vi "Main2000.vi"() -> ()   [LabVIEW 2016]
doc: "Use this template to create an application that executes until you click the Stop button. Unlike the Single Loop Application VI that uses polling, this VI uses the Event Structure."
uses:
  <vilib>/vision/driver/NI_Vision_Acquisition_Software.lvlib
  <vilib>/vision/NI_Vision_Development_Module.lvlib
  Granule-2000AT/PC/llb/Library.lvlib
  <vilib>/Utility/file.llb/Write To Spreadsheet File (string).vi
  <vilib>/Utility/file.llb/Read From Spreadsheet File (string).vi
  <vilib>/userdefined/High Color/IMAQdx.ctl
panel:
  in  "Arhive":bool
  in  "M_PLasmatron":dbl
  out "V барабаны 2":dbl
  in  "Tab Control 2":enum32{"X1", "X2", "Y"}(tab)
  out "X240":bool[](array[boolean])
  out "ОП1 Х1 5":string[](array[string])
  out "X200":bool[](array[boolean])
  out "ОП1 Х1 4":string[](array[string])
  out "X140":bool[](array[boolean])
  out "ОП1 Х1 3":string[](array[string])
  out "X100":bool[](array[boolean])
  out "ОП1 Х1 2":string[](array[string])
  out "X400":bool[](array[boolean])
  out "ОП1 Х1 8":string[](array[string])
  out "X340":bool[](array[boolean])
  out "ОП1 Х1 7":string[](array[string])
  out "X300":bool[](array[boolean])
  out "ОП1 Х1 6":string[](array[string])
  out "Y120":bool[](array[boolean])
  out "ОП1 Х1 10":string[](array[string])
  out "Y60":bool[](array[boolean])
  out "ОП1 Х1 9":string[](array[string])
  out "Air 4":bool
  in  "PT3 2":dbl
  in  "Запись отчета":bool
  out "V вращ. бараб 2":string caption="V заготовки"
  out "LONGITUDINAL SPEED":string
  out "PLASMATRON SPEED":string
  in  "mac3":bool
  in  "Ошибка 2":i16 format="%x"
  in  "Скорость пп 2":i16
  out "Полож заг сер":bool
  out "Полож заг нач":bool caption="НАЧАЛО"
  out "Полож заг кон":bool
  out "Полож плазм кон":bool caption="Конец"
  out "Полож плазм сер":bool caption="Пром."
  out "Полож плазм  нач":bool caption="Начало"
  in  "МАКСИМАЛЬНАЯ СКОРОСТЬ ПП К":bool
  in  "v4066_cкорость подачи плазматрона":dbl
  in  "v4065_cкорость подачи":dbl
  in  "V7045_I_ist":dbl
  in  "V7045_U_ist":dbl
  in  "Действующий ток на плазматроне":string caption="Ток А"
  out "V заготовки":string
  in  "D, заготовки":i16
  in  "Закончить автораспыление":bool
  in  "Автораспыление доплавить":bool
  in  "Автораспыление начать":bool
  in  "задание тока А":string caption="Задание, А"
  in  "ПОДАЧА ЗАГОТОВКИ":bool
  in  "stop 3":bool
  in  "stop 2":bool
  in  "SP_зазор":dbl
  in  "PV_зазор":dbl
  in  "max out":dbl
  in  "out":dbl
  out "Distance зазор":sgl format="%.2f"
  out "x/y":dbl
  out "x*y":dbl
  out "16bit integer":i16
  in  "Numeric":i16
  in  "Т6":dbl
  in  "Улавливатель закрыть":bool
  in  "Улавливатель открыть":bool
  in  "Ролик прижать":bool
  in  "Ролик отжать":bool
  in  "PE3":dbl
  in  "PE2":dbl
  in  "PE1":dbl
  in  "ЗАДАНИЕ ТОКА":i16
  in  "ГС - Закрыть":bool
  in  "ГС -Открыть":bool
  out "ГС - Плазматрон":string caption="Плазматрон"
  out "ГС - Камера":string caption="Камера"
  in  "Скорость пп":i16
  in  "V барабаны задание":dbl
  in  "Выход":bool
  in  "ГС ПТ":i16
  in  "ГС камера":i16
  in  "V барабаны":dbl
  in  "Т5":dbl
  in  "Т4":dbl
  in  "Т3":dbl
  in  "Т2":dbl
  in  "Т1":dbl
  in  "Ошибка":i16
  in  "PT3":dbl
  in  "PT2":dbl
  in  "PT1":dbl
  in  "y120":i32
  in  "y60":i32
  in  "x400":i32
  in  "x340":i32
  in  "x300":i32
  in  "x240":i32
  in  "x200":i32
  in  "x140":i32
  in  "x100":i32
  in  "Tab Control":enum32{"VACUUM", "WORK", "INPUTS"}(tab)
  in  "forvacuum":bool
  in  "forvakuum led":bool
  in  "Slide":dbl(slide) scale=0.0..99.0
  out "PD2":u16(ring)
  out "NL 2":u16(ring)
  out "VP6":u16(ring)
  in  "ND HEAT BUT":bool
  in  "ND HEAT LED":bool
  in  "откачка стоп 2":bool
  in  "откачка стоп индик 2":bool
  out "Water-2":bool
  out "Water-1":bool
  out "Air":bool
  out "PT 4":string caption="Вакуум в камере\nPT2 (torr)"
  in  "откачка стоп":bool
  in  "откачка стоп индик":bool
  out "EV1":u16(ring)
  out "EV2":u16(ring)
  out "EV3.3":u16(ring)
  out "EV3.2":u16(ring)
  out "PE2":u16(ring)
  out "PE2":string caption="Вакуум в камере\nPT2 (torr)"
  out "CO1":u16(ring)
  out "CO2":u16(ring)
  out "EV3.1":u16(ring)
  out "CO3":u16(ring)
  out "P1":u16(ring)
  out "PE1":u16(ring)
  out "PE1":string caption="Вакуум в камере\nPT2 (torr)"
  out "PE3":u16(ring)
  out "PE3":string caption="Вакуум в камере\nPT2 (torr)"
  out "VP1":u16(ring)
  out "VP2":u16(ring)
  out "PT3":u16(ring)
  out "PT2":u16(ring)
  out "PT 2":string caption="Вакуум в камере\nPT2 (torr)"
  out "VP3":u16(ring)
  out "VP5":u16(ring)
  out "PD1":u16(ring)
  out "PT1":u16(ring)
  out "PT 1":string caption="Вакуум в камере\nPT2 (torr)"
  out "NZ":u16(ring)
  out "NB":u16(ring)
  out "NL":u16(ring)
  out "VP4":u16(ring)
  in  "mac 4":bool
  in  "напустить аргон":bool
  in  "откачать рабочий вакуум":bool
  in  "mac 2":bool
  out "PT 3":string caption="Вакуум в камере\nPT2 (torr)"
  out "УГ_закрыт":bool caption="Close"
  out "УГ_открыт":bool caption="Open"
  out "ролик_отжат":bool caption="Up"
  out "ролик_прижат":bool caption="Down"
  out "max Speed":string caption="Max speed (r/min)"
  out "ТЕМП КАМЕРА":string caption="T gas (C°)"
  in  "Скорость ПП 2":string caption="Plasmatron speed (mm/min)"
  in  "Скорость ПП":string caption="Longitudial speed (mm/min)"
  out "ТЕМП РОЛИК":string caption="T roller (C°)"
  out "ПОДШ. 2.2":string caption="T4 (C°)"
  out "ПОДШ. 2.1":string caption="T3 (C°)"
  out "ПОДШ. 1.2":string caption="T2 (C°)"
  out "ПОДШ. 1.1":string caption="T1 (C°)"
  out "P plasmatron (bar)":string
  out "P camera (bar)":string
  out "I_ist":string caption="Current (A)"
  out "U_ist":string caption="Voltage (V)"
  in  "Tab Control 3":enum32{"PARAMETERS VIDEO", "RID"}(tab)
  in  "Media Stop Button":bool
  in  "Play Button":bool
  in  "CAM":T1
  in  "HOOK":T2 {"Rotation" format="%.2f"; "Left" scale=0.0..1024.0; "Right" scale=0.0..1280.0}
  in  "PARAMETERS VIDEO":T3={"Contrast"=40, "Filter width"=4, "Steepness"=2, "Subsampling Ratio"=5, "Show Search Area"=FALSE, "Show Search Lines"=FALSE, "Show Edges Found"=FALSE, "Show Result"=TRUE}
  in  "WORK COLOR":u32(colorbox)
  in  "CALIBRATION":u32(colorbox)
  in  "DELAY":u32
  in  "BINAR LEVEL":cluster{"DOWN LEVEL":sgl, "UP LEVEL":sgl}={"DOWN LEVEL"=128.0, "UP LEVEL"=255.0} {"UP LEVEL" format="%.2f"; "DOWN LEVEL" format="%.2f"}
  in  "SHEMA":i32(ring)=1 items=["Red", "Green", "Blue", "Hue", "Saturation", "Luminance", "Value", "Intensity"]
  out "Индикатор камеры":bool
  in  "Blank Button":bool
  out "Индикатор камеры 2":bool
  in  "Сохранить настройки":bool
  out "String":string
  out "Record":bool
  out "Максимальная подача (мм/мин)2":string caption="Max speed\n(mm/min)"
  out "Boolean":bool
  in  "Регулятор":bool caption="RID"
  out "Actual speed\n(mm/min)":string
  out "PV(mm)":string
  out "SP (mm)":string
  in  "взять зазор":bool caption="Регулятор"
  out "Марка сплава":string caption="Mark"
  out "Порядковый номер":string caption="Billet number (un)"
  in  "Position (mm)":dbl(slide) scale=0.0..820.0
  out "Диаметр заг.":string caption="Diameter (mm)"
  out "V задания":string caption="Rotation speed (r/min)"
  out "V вращ. бараб":string caption="Rotation frequency (r/min)"
  in  "ЗУ-вверх":bool
  out "ИНдикатор положения полки":string
  in  "Продол впер":bool
  in  "Продол назад":bool
  in  "ПЛАЗМАТРОН В ИСХОДНОЕ":bool
  out "индикация видео":T4(plugin-control)
  in  "ПЛАЗМАТРОН В ИСХОДНОЕ 2":bool
  out "PULLEYS":dbl(graph)
  out "PV":dbl(graph)
  out "LONGITUDINAL FEED":dbl(graph)
  out "CURRENT":dbl(graph)
  out "VOLTAGE":dbl(graph)
  out "voto plasmatron":string caption="MOTO\nPLASMATRON"
  out "текущее время":string
  # "Ролик"
  # "Улавливатель ОГ"
  # "Обработка"
  # "БАРАБАНЫ"
  # "РАСПЫЛЕНИЕ ЗАГОТОВКИ"
  # "Температура"
  # "3A3.1 X100-X137"
  # "3A3.2 X140-177"
  # "3A4 X200-X237"
  # "3A5.1 X240-X277"
  # "3A5.2 X300-X337"
  # "3A6 X340-X377"
  # "3A8 X400-X437"
  # "2A8 Y60-Y117"
  # "3A7 Y120-Y157"
  # "Положение толкателя"
  # "Положение плазматрона"
  # "Газовая система"
  # "VF1"
  # "Ar,He"
  # "PC1"
  # "PC2"
  # "SYSTEM"
  # "PLASMATRON"
  # "CATCHER CINDERS"
  # "PINCH ROLLER"
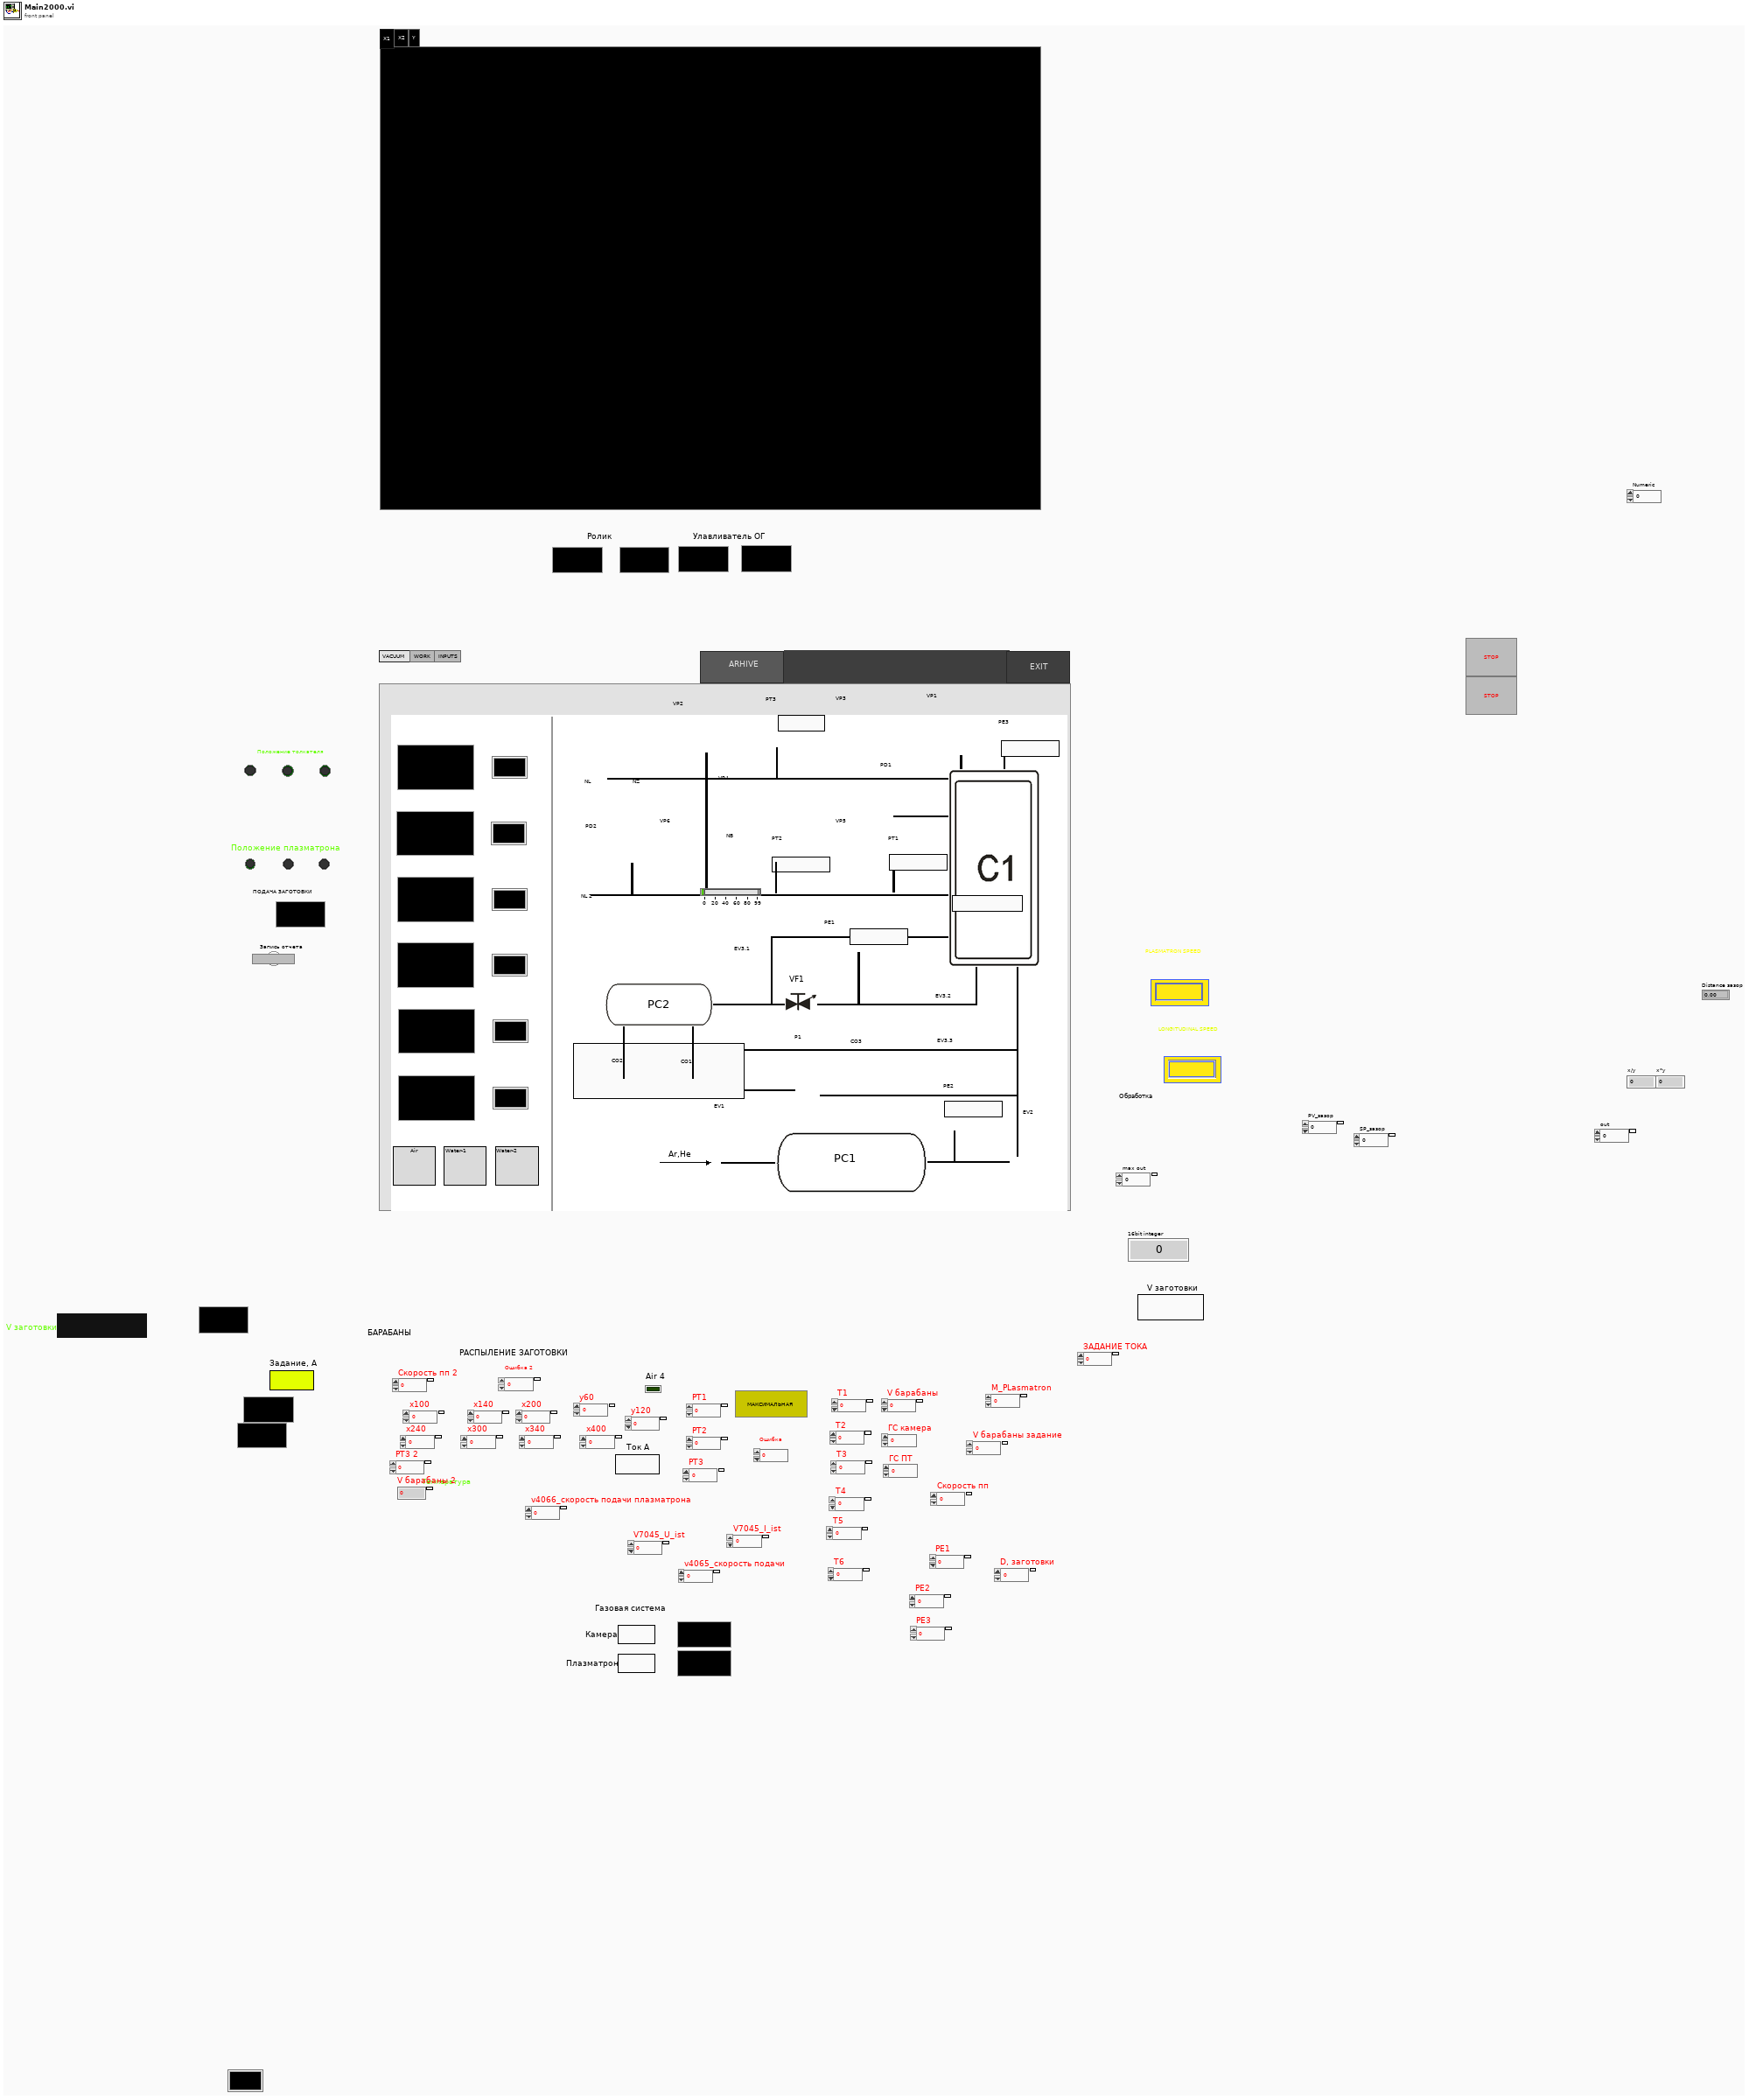
[diagram p1: front panel]
types:
  T1 = typedef "Library.lvlib/IMAQdx.ctl" = refnum<k21>
  T2 = typedef "IMAQ Rectangle" = cluster{"Left":i32, "Top":i32, "Right":i32, "Bottom":i32, "Rotation":dbl}
  T3 = cluster{"Contrast":i32, "Filter width":i32, "Steepness":i32, "Subsampling Ratio":u32, "Show Search Area":bool, "Show Search Lines":bool, "Show Edges Found":bool, "Show Result":bool}
  T4 = typedef "IMAQ Image.ctl" = refnum<image>
  T5 = enum16{"open", "replace", "create", "open or create", "replace or create", "replace or create with confirmation"}
  T6 = enum8{"Enabled", "Disabled", "Disabled and Grayed Out"}
  T7 = cluster{i32, i32, i32, u32, "Boolean":bool, "Boolean":bool, "Boolean":bool, "Boolean":bool}
  T8 = typedef "Image Type" = u32
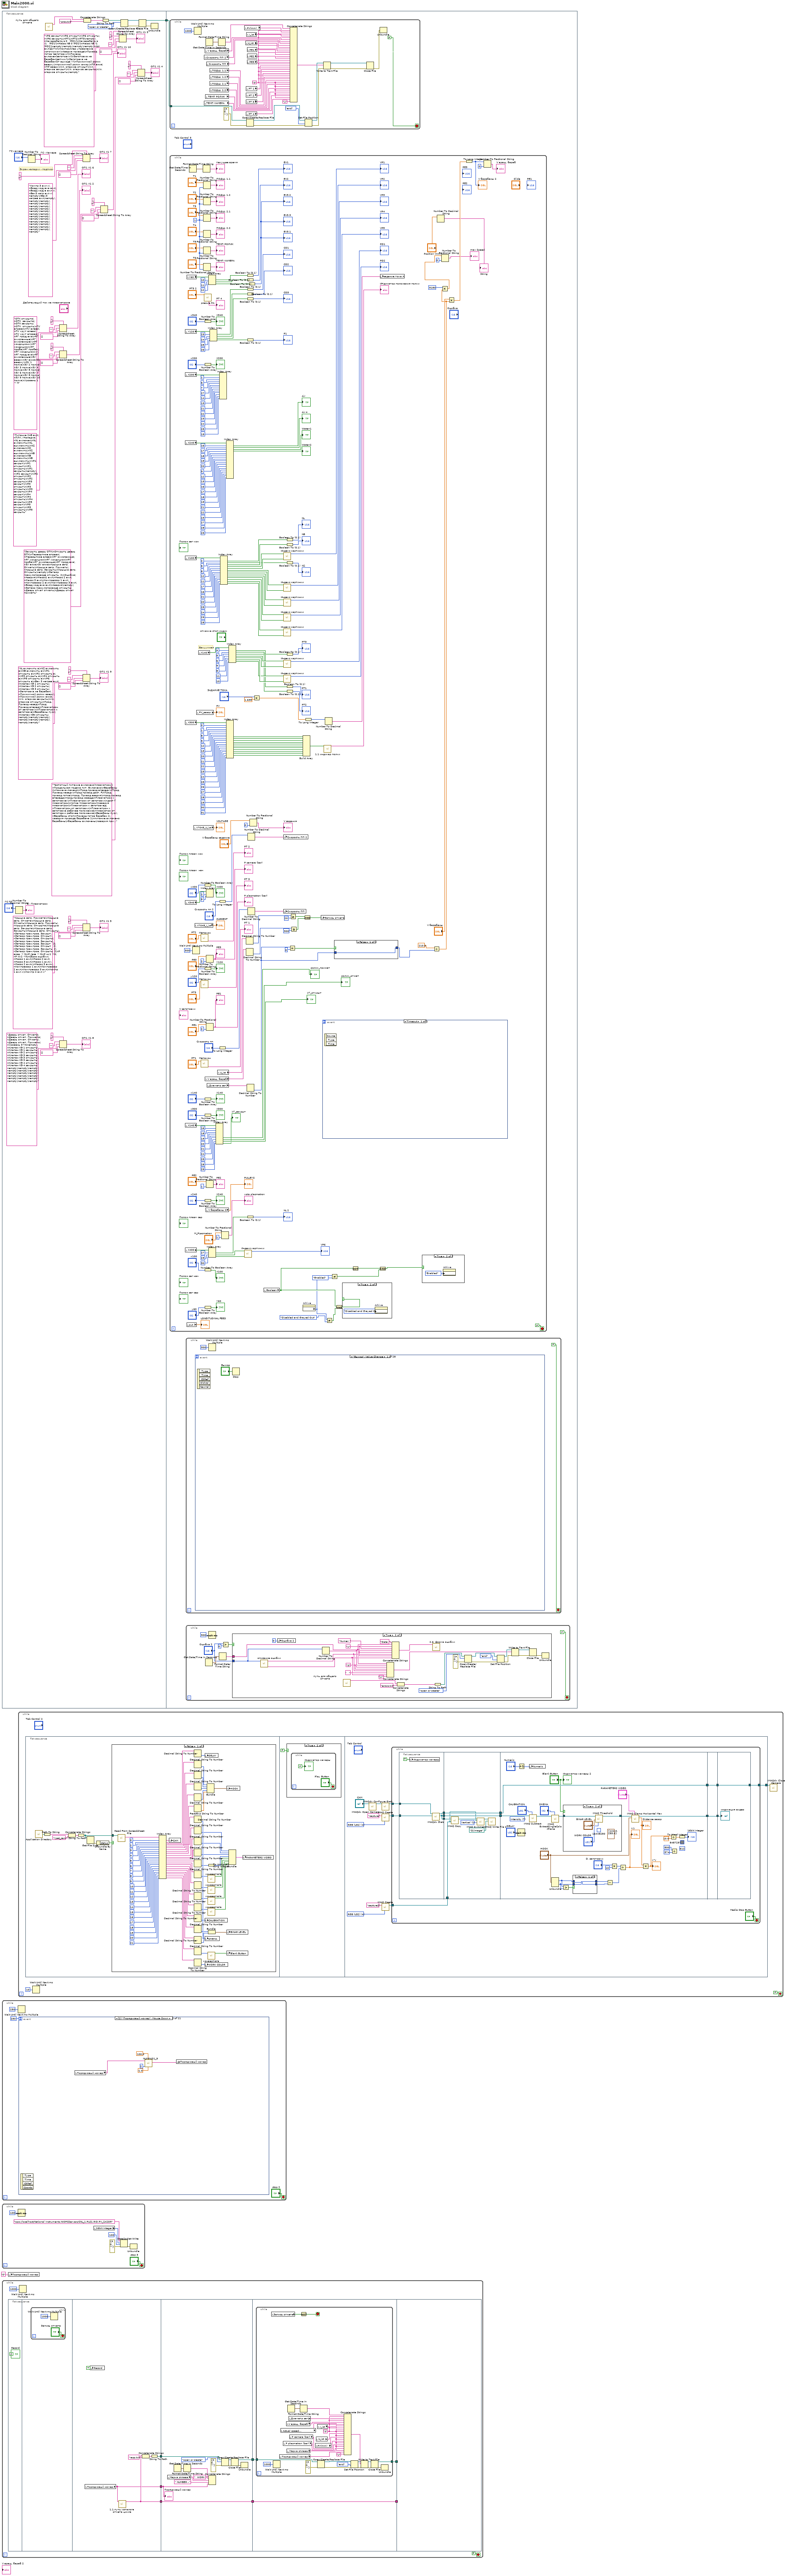
[diagram p0: block diagram]
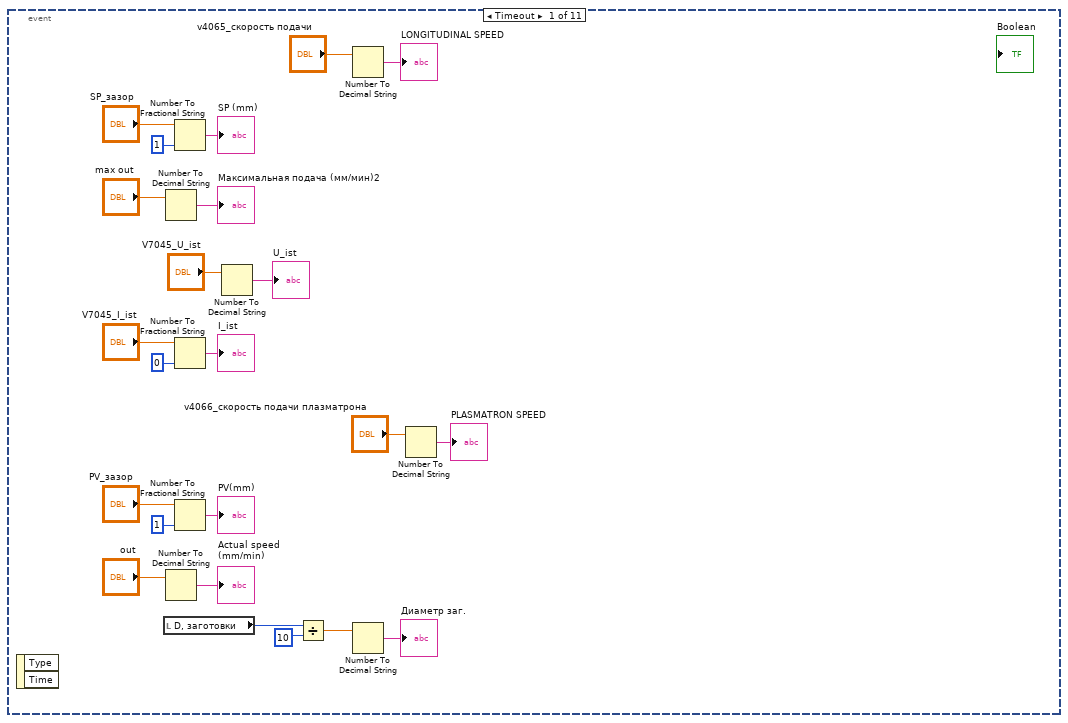
[diagram p6: hidden frame]
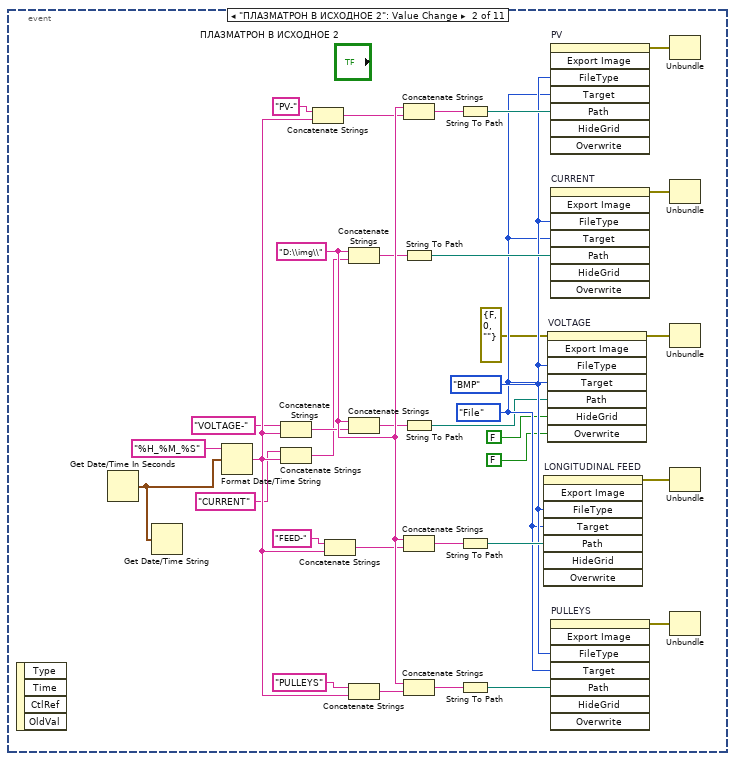
[diagram p7: hidden frame]
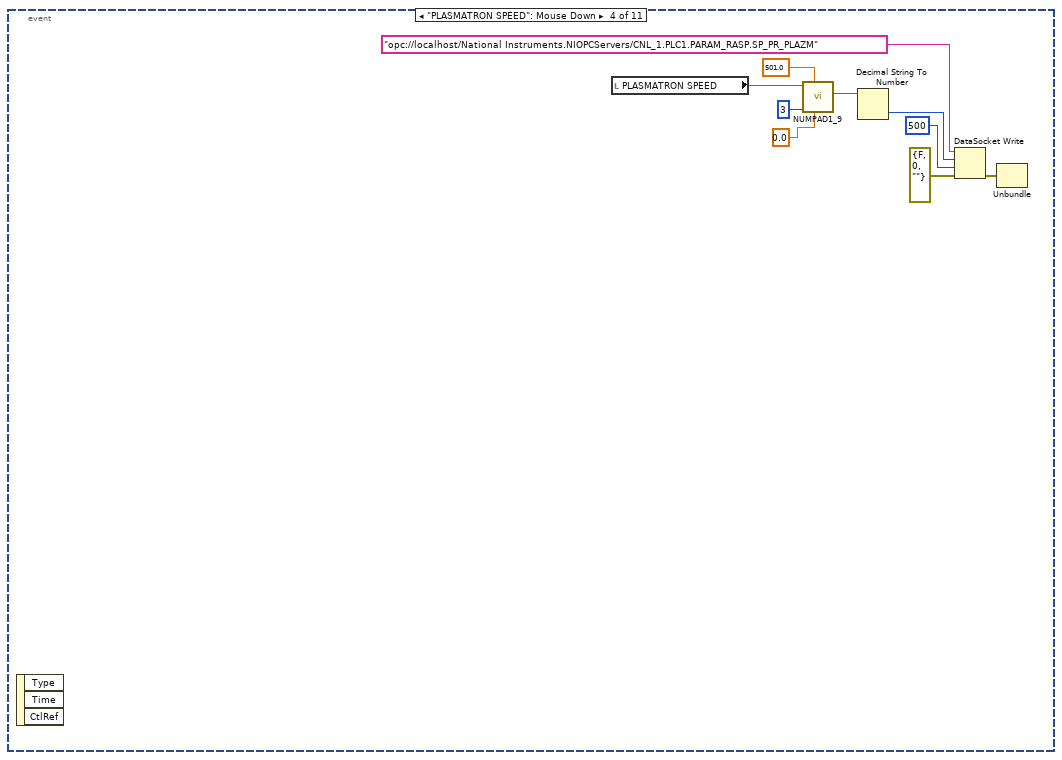
[diagram p8: hidden frame]
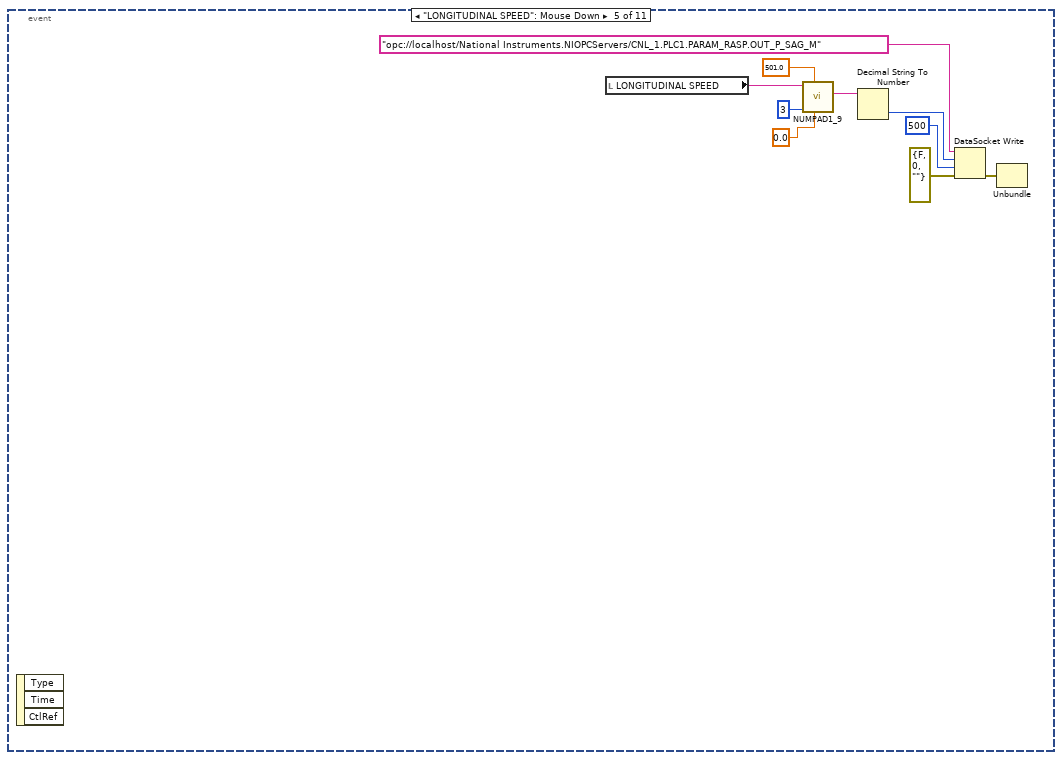
[diagram p9: hidden frame]
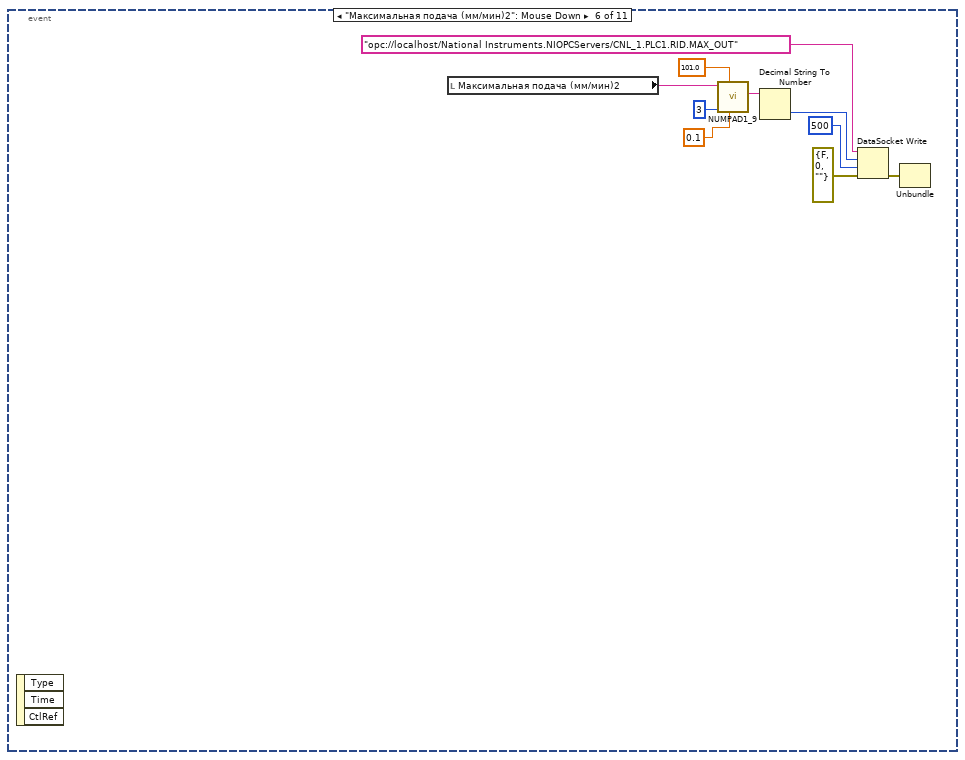
[diagram p10: hidden frame]
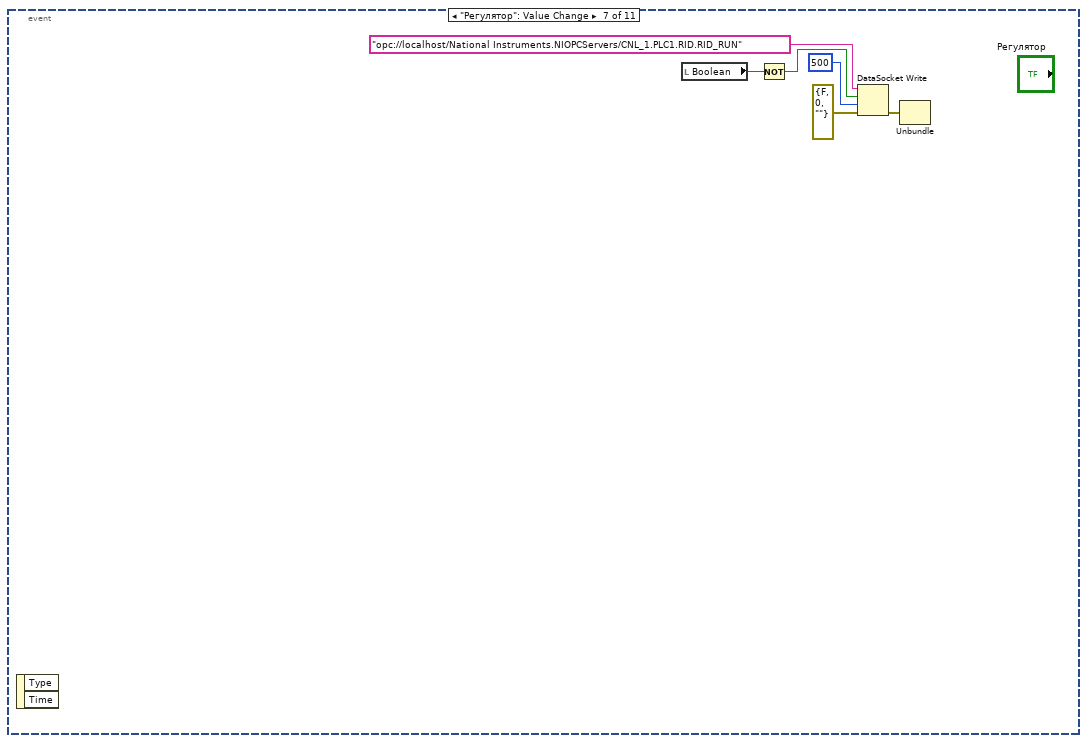
[diagram p11: hidden frame]
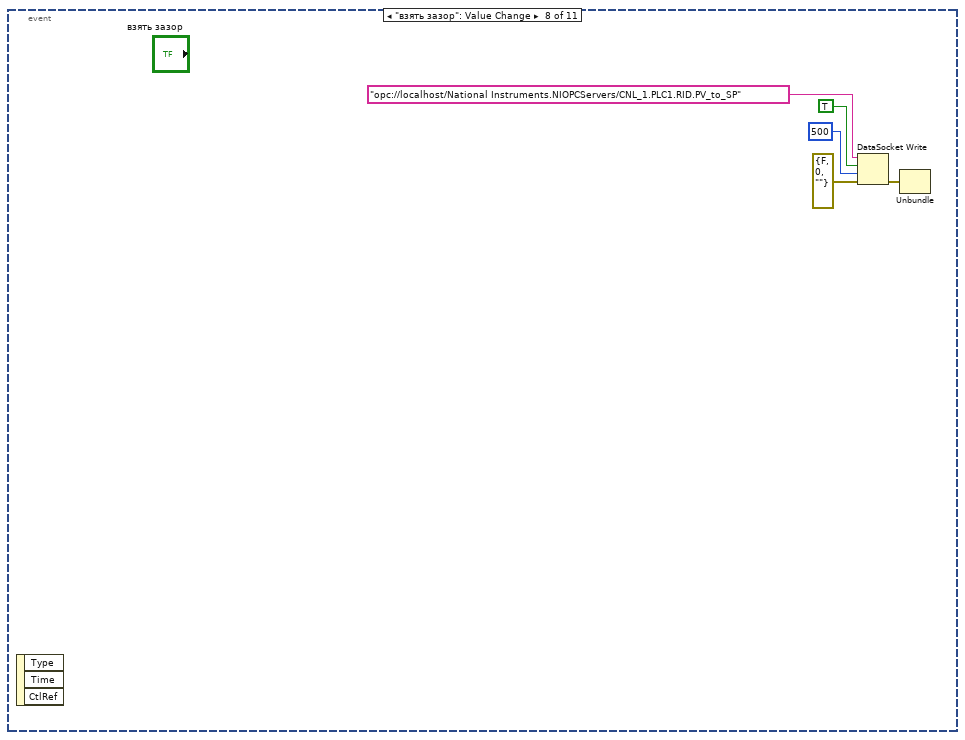
[diagram p12: hidden frame]
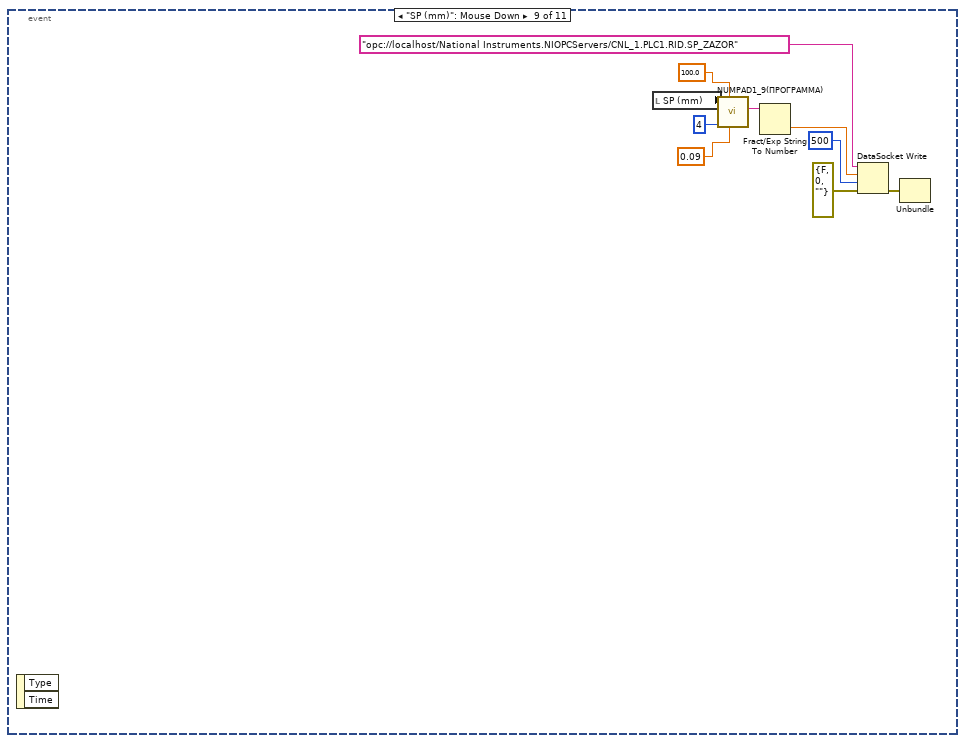
[diagram p13: hidden frame]
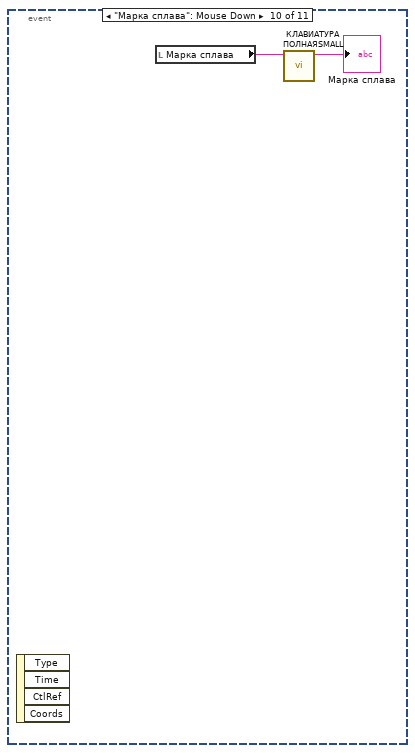
[diagram p14: hidden frame]
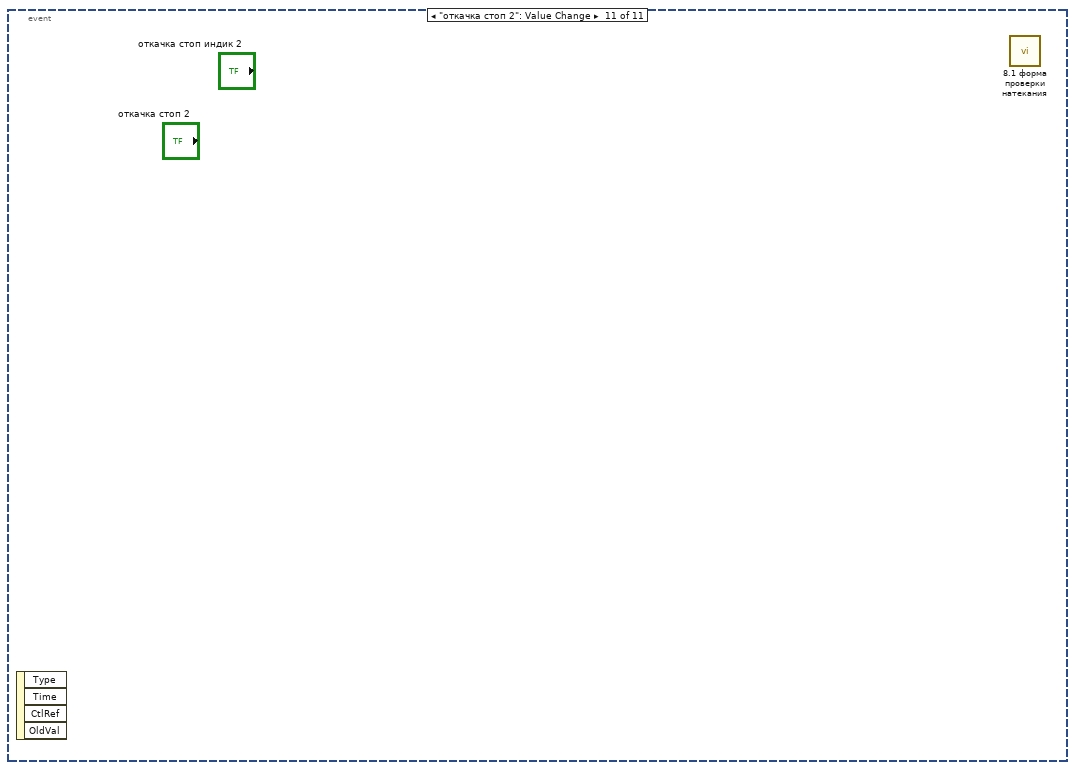
[diagram p15: hidden frame]
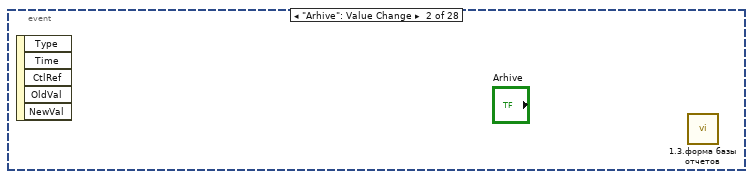
[diagram p17: hidden frame]
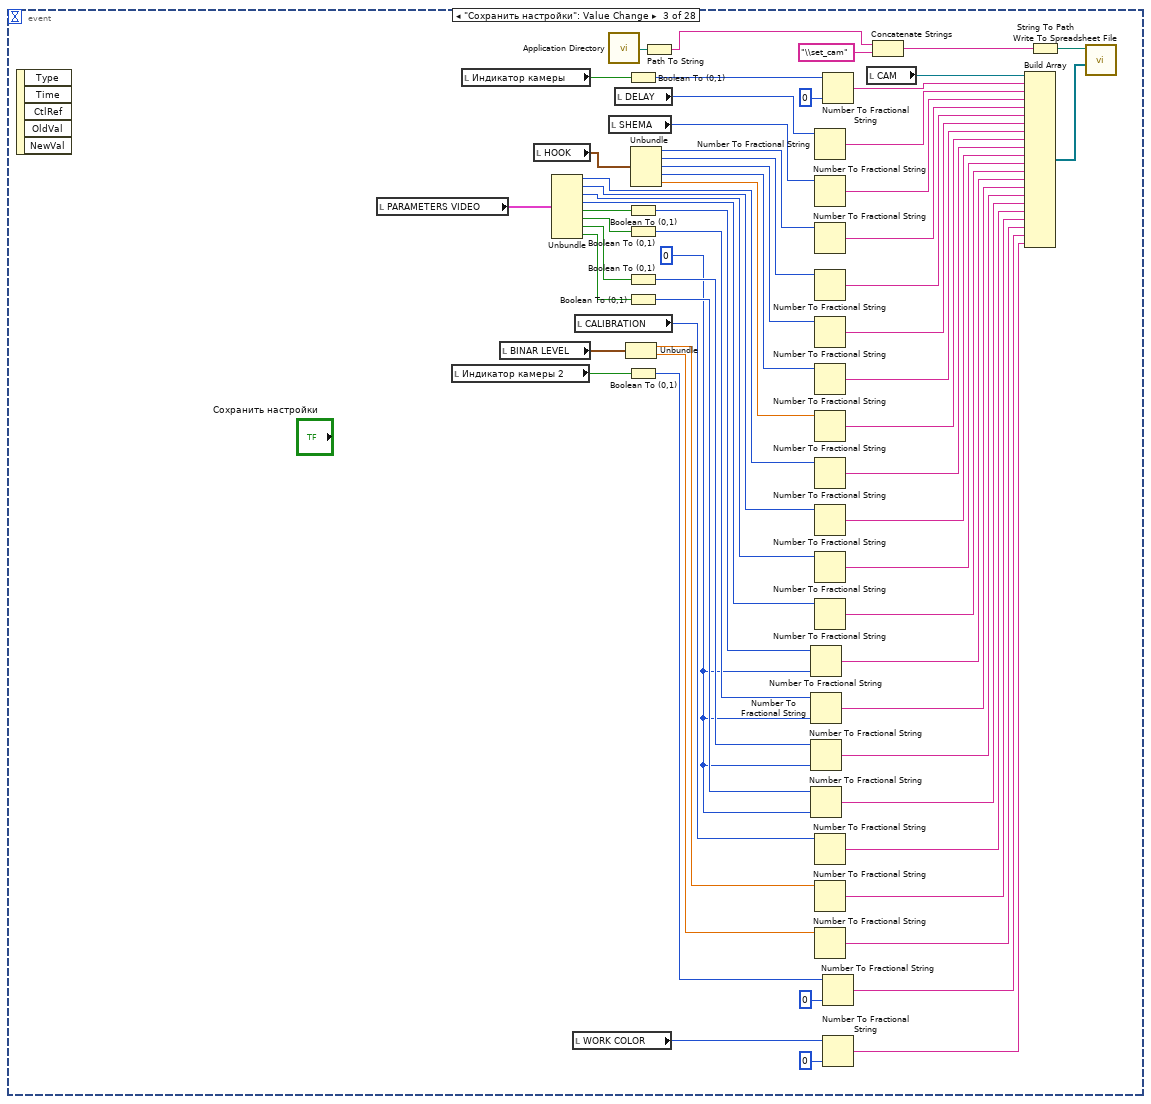
[diagram p18: hidden frame]
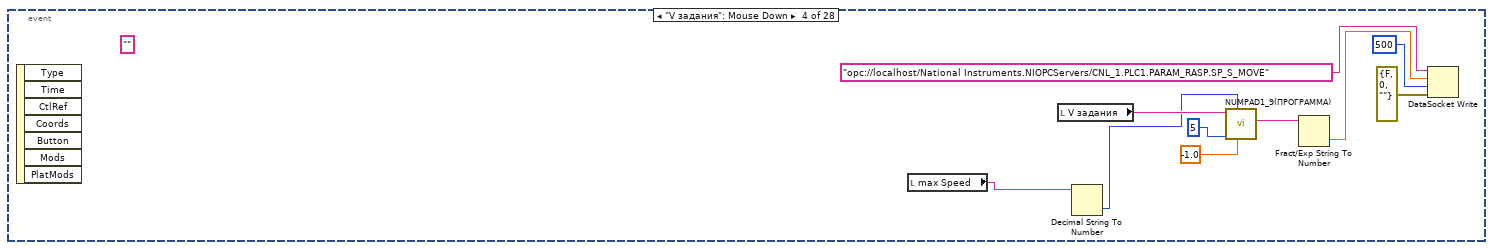
[diagram p19: hidden frame]
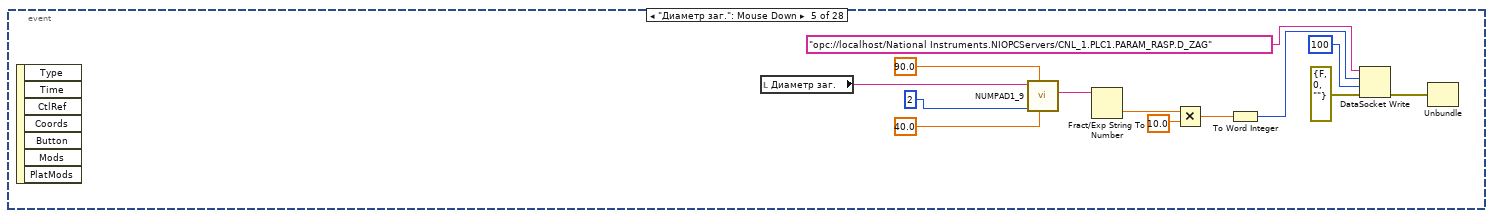
[diagram p20: hidden frame]
diagram:
  n1 = flat-sequence {
    tunnel: [w3] -> w1
    tunnel: w1 -> [w61]
    frame #0 {
      # "Экран наладки - подписи"
      n2 = Number To Decimal String(number="ГС ПТ") -> (decimal integer string=→"ГС - Плазматрон":string)  [unwired: 1 in]
      n3 = Number To Decimal String(number="ГС камера") -> (decimal integer string=→"ГС - Камера":string)  [unwired: 1 in]
      n4 = call "путь для общего отчета.vi"() -> ("path_out 2"=w9:string)  [unwired: 11 in]
      n5 = Spreadsheet String To Array(delimiter (Tab)="\n", format string="", spreadsheet string="ОТК открыта\nОТК  закрыта\nОТК закрыть\nОТК  открыть\nПУ вправо\nПУ влево\nПУ крут влево\nПУ крут вправо\nРГ продувка\nРГ окисленные\nРГ окисленныек\nРГ кондиционк\nРГ кондицион\nРГ проба\nРГ пробак\nРГ кондиционкк\nРГ продувка\nРГ окисленные\nЗУ вверх\nЗУ вниз\nЗУ вверху\nЗУ 1 полка\nЗУ 2 полка\nЗУ 3 полка\nЗУ 4 полка\nЗУ 5 полка\nЗУ 6 полка\nЗУ 7 полка\nЗУ 8 полка\nЗУ 9 полка\nЗУ 10 полка\nУровень 1 < N", array type (2D Dbl)=string[] [] ("ОП1 Х1")) -> (array=→"ОП1 Х1 6":string[])
      n6 = Spreadsheet String To Array(delimiter (Tab)="\n", format string="", spreadsheet string="Питание 24В вкл\nПЛК / Наладка\nNL включен\nNL включить\nNL выключить\nNZ включен\nNZ включить\nNZ выключить\nNB включен\nNB включить\nNB выключить\nVP1 закрыт\nVP1 открыт\nVP1 открыть\nVP1 закрыть\nempty\nVP2 закрыт\nVP2 открыт\nVP2 открыть\nVP2 закрыть\nVP3 закрыт\nVP3 открыт\nVP3 открыть\nVP3 закрыть\nVP4 закрыт\nVP4 открыт\nVP4 открыть\nVP4 закрыть\nVP5 закрыт\nVP5 открыт\nVP5 открыть\nVP5 закрыть", array type (2D Dbl)=string[] [] ("ОП1 Х1")) -> (array=→"ОП1 Х1 2":string[])
      n7 = Spreadsheet String To Array(delimiter (Tab)="\n", format string="", spreadsheet string="Дверь откат. Отжата\nДверь откат. Прижата\nДверь откат. Отжать\nДверь откат. Прижать\nУровень 3<N\nempty\nКлапан КЭ 1 открыть\nКлапан КЭ 1 закрыть\nКлапан КЭ 2 открыть\nКлапан КЭ 3 закрыть\nКлапан КЭ 3 открыть\nКлапан КЭ 3 закрыть\nКлапан КЭ 4 открыть\nКлапан КЭ 4 закрыть\nempty\nempty\nempty\nempty\nempty\nempty\nempty\nempty\nempty\nempty\nempty\nempty\nempty\nempty\nempty\nempty\nempty\nempty", array type (2D Dbl)=string[] [] ("ОП1 Х1")) -> (array=→"ОП1 Х1 8":string[])
      n8 = Spreadsheet String To Array(delimiter (Tab)="\n", format string="", spreadsheet string="Компр 3 вкл к\nВоздуходувка вкл\nВоздуходув вкл к\nБак3 нагр вкл к\nempty\nБак3 нагрев вкл\nempty\nempty\nempty\nempty\nempty\nempty\nempty\nempty\nempty\nempty\nempty\nempty\nempty\nempty\nempty\nempty\nempty\nempty\nempty\nempty\nempty\nempty\nempty\nempty\nempty\nempty", array type (2D Dbl)=string[] [] ("ОП1 Х1")) -> (array=→"ОП1 Х1 7":string[])
      n9 = Spreadsheet String To Array(delimiter (Tab)="\n", format string="", spreadsheet string="NL включить в\nNZ включить в\nNB включить в\nVP1 открыть в\nVP2 открыть в\nVP3 открыть в\nVP4 открыть в\nVP5 открыть в\nVP6 открыть в\nБак 3 нагрев вкл\nКлапан КЭ 1 открыть\nКлапан КЭ 2 открыть\nКлапан КЭ 3 открыть\nЗаготовка на барабан\nПрижимной ролик вверх\nПрижимной ролик вниз\nУл. огарков закрыть\nУл. огарков открыть\nПрод. Привод назад\nПрод. Привод вперед\nПлазматрон от заготовки\nПлазматрон к заготовке\nБарабаны пуск\nКлапан КЭ4 открыть\nempty\nempty\nempty\nempty\nempty\nempty\nempty\nempty", array type (2D Dbl)=string[] [] ("ОП1 Х1")) -> (array=→"ОП1 Х1 9":string[])
      n10 = Spreadsheet String To Array(delimiter (Tab)="\n", format string="", spreadsheet string="Крышка загр. Прижата\nКрышка загр. Отжата\nКрышка загр. Отжать\nКрышка загр. Прижать\nКрышка загр. Открыта\nКрышка загр. Закрыта\nКрышка загр. Закрыть\nКрышка загр. Открыть\nЗатвор гран.пров. Закрыт\nЗатвор гран.пров. Открыт\nЗатвор гран.пров. Открыть\nЗатвор гран.пров. Закрыть\nЗатвор гран.пров. Закрыт   2\nЗатвор гран.пров. Открыт   2\nЗатвор гран.пров. Закрыть  2\nЗатвор гран.пров. Открыть  2\nP возд. < N\nP газа < N\nP нк1 <N\nP нк2 <N\nСброс ошибки\nНасос 1 вкл\nНасос 2 вкл\nНасос 3 вкл\nНасос 1 вклк\nНасос 2 вклк\nНасос 3 вклк\nКомпрессор 1 вкл\nКомпрессор 2 вкл\nКомпрессор 3 вкл\nКомпр 1 вкл к\nКомпр 2 вкл к", array type (2D Dbl)=string[] [] ("ОП1 Х1")) -> (array=→"ОП1 Х1 5":string[])
      n11 = Concatenate Strings(w9, "proc.txt") -> (w11:string)
      n12 = Spreadsheet String To Array(delimiter (Tab)="\n", format string="", spreadsheet string="Закрыть дверь ОТК\nОткрыть дверь ОТК\nПересыпное вправо\nПересыпное влево\nРГ окисленные\nРГ кондицион\nРГ кондицион\nРГ проба\nРГ окисленные\nРГ продувка\nЗУ вниз\nЗУ вниз\nКрышка загр. Отжать\nКрышка загр. Прижать\nКрышка загр. Закрыть\nКрышка загр. Открыть\nempty\nЗатвор гранулопровода открыть  2\nОшибка\nАвария\nНасос1 вкл\nНасос 2 вкл\nНасос 3 вкл\nКомпрессор 1 вкл\nКомпрессор 2 вкл\nКомпрессор 3 вкл\nВоздуходувка вкл\nАвария\nempty\nЗатвор гранулопровода открыть\nДверь откат отжать\nДверь откат прижать", array type (2D Dbl)=string[] [] ("ОП1 Х1")) -> (array=→"ОП1 Х1 10":string[])
      n13 = String To Path(string=w11) -> (path=w7:path)
      n14 = Spreadsheet String To Array(delimiter (Tab)="\n", format string="", spreadsheet string="VP6 закрыт\nVP6 открыт\nVP6 открыть\nVP6 закрыть\nPT1\nPT2\nPT3\nempty\nКамераЗагруз 0   (PD1)\nКамераЗагруз -1   (PD1)\nНасос NB 0 (PD2)\nНасос NB -1 (PD2)\nempty\nempty\nempty\nempty\nИст вкл(ДУГА)\nКонтроллер управление источником\nАвария привода\nПривод готов (заготовки)\nПривод включен(заготовки)\nЗаготовка на барабан(датчик)\nЗаготовка на барабан(от выхода Y)\nПрижимной ролик вверху\nприжимной ролик внизу\nПР вниз\nПР вверх\nУл. огарков открыт\nУл. огарков закрыт\nУл. огарков закрыть\nУл. огарков открыть\nempty", array type (2D Dbl)=string[] [] ("ОП1 Х1")) -> (array=→"ОП1 Х1 3":string[])
      n15 = Open/Create/Replace File(file path (use dialog)=w7, operation (0:open)=T5."open or create") -> (refnum out=w4:refnum<file>, error out=w5:errorcluster)  [unwired: 4 in, 1 out]
      n16 = Spreadsheet String To Array(delimiter (Tab)="\n", format string="", spreadsheet string="Частотный питание включено(плазматрон)\nПродольная подача пит. Включено\nБарабаны питание включено\nПрод.привод впередк\nПрод. Привод назадк\nПрод привод дост. F\nПрод.привод готов\nпрод. Привод авария\nпрод.привод впередд\nпрод.привод назадд\nПлазматрон к заготовкек\nПлазматрон от заготовки\nдост f   плазматрон\nготов (плазматрон)\nавария плазматрон\nПлазматрон к заготовкед\nПлазматрон от заготовки\nПлазматрон к заготовке рабочее положение\nплазматро от заготовки рабочее положение\nБарабаны пуск\nБарабаны стоп\nПривод готов барабан 1\nавария привода барабана 1\nпитание включено барабаны\nбарабаны включены\nавария привода барабана 2\nпривод готов барабан 2\nПеремещение плазматрона пит. Включено\nempty\nПрижимной ролик вверху\nПрижимной ролик внизу\nempty", array type (2D Dbl)=string[] [] ("ОП1 Х1")) -> (array=→"ОП1 Х1 4":string[])
      n17 = Close File(refnum=w4, error in=w5) -> (path=w3:path, error out=w8:errorcluster)
      n18 = Unbundle(w8) -> ()  [unwired: 3 out]
    }
    frame #1 {
      n19 = while {
        tunnel: w61 -> [w88]
        stop <- FALSE stop-if-true
        w64 = "\t"
        n20 = Wait Until Next ms Multiple(millisecond multiple=u32 1000 ("milliseconds to wait")) -> ()  [unwired: 1 out]
        n21 = local read "Скорость ПП 2"() -> (w82:string)
        n22 = local read "ТЕМП КАМЕРА"() -> (w65:string)
        n23 = local read "V вращ. бараб"() -> (w83:string)
        n24 = local read "ТЕМП РОЛИК"() -> (w71:string)
        n25 = Get Date/Time In Seconds() -> (seconds since 1Jan1904=w97:timestamp)
        n26 = local read "Скорость ПП"() -> (w81:string)
        n27 = local read "ПОДШ. 1.1"() -> (w69:string)
        n28 = local read "ПОДШ. 1.2"() -> (w74:string)
        n29 = local read "ПОДШ. 2.1"() -> (w73:string)
        n30 = local read "ПОДШ. 2.2"() -> (w72:string)
        n31 = Format Date/Time String(seconds (now)=w97) -> (date/time string=w66:string)  [unwired: 2 in]
        n32 = local read "PV(mm)"() -> (w67:string)
        n33 = local read "U_ist"() -> (w80:string)
        n34 = local read "PT 1"() -> (w76:string)
        n35 = local read "PT 2"() -> (w75:string)
        n36 = local read "PT 3"() -> (w70:string)
        n37 = local read "PT 4"() -> (w63:string)
        n38 = local read "I_ist"() -> (w68:string)
        n39 = Open/Create/Replace File(file path (use dialog)=w88, error in=errorcluster {"status"=FALSE, "code"=0, "source"=""}) -> (refnum out=w96:refnum<file>, error out=w94:errorcluster)  [unwired: 4 in, 1 out]
        n40 = local read "PE1"() -> (w79:string)
        n41 = local read "PE2"() -> (w78:string)
        n42 = local read "PE3"() -> (w77:string)
        n43 = Concatenate Strings(w66, w64, w67, w64, w68, w64, w83, w64, w82, w64, w81, w64, w80, w64, w79, w64, w78, w64, w77, w64, w76, w64, w75, w64, w70, w64, w69, w64, w74, w64, w73, w64, w72, w64, w71, w64, w65, w64, w63, "\r") -> (w86:string)
        n44 = Set File Position(refnum=w96, from (0:start)=enum16{"start", "end", "current"}."end", error in=w94) -> (refnum out=w93:refnum<file>, error out=w92:errorcluster)  [unwired: 1 in]
        n45 = Write to Text File(file (use dialog)=w93, text=w86, error in=w92) -> (refnum out=w91:refnum<file>, error out=w90:errorcluster)  [unwired: 1 in, 1 out]
        n46 = Close File(refnum=w91, error in=w90) -> (error out=w89:errorcluster)  [unwired: 1 out]
        n47 = Unbundle(w89) -> ()  [unwired: 3 out]
      }
      n48 = while {
        stop <- FALSE stop-if-true
        w394 = i16 1 ("precision (6)")
        # "Вакуумная"
        n49 = local read "Y120"() -> (w544:bool[])
        n50 = local read "X200"() -> (w606:bool[])
        n51 = local read "X240"() -> (w590:bool[])
        n52 = local read "X100"() -> (w410:bool[])
        n53 = local read "X300"() -> (w565:bool[])
        n54 = local read "X340"() -> (w551:bool[])
        n55 = local read "X140"() -> (w625:bool[])
        n56 = local read "X400"() -> (w473:bool[])
        n57 = local read "Y60"() -> (w545:bool[])
        n58 = local read "out"() -> (→"LONGITUDINAL FEED":dbl)
        n59 = Get Date/Time In Seconds() -> (seconds since 1Jan1904=w483:timestamp)
        n60 = Wait Until Next ms Multiple(millisecond multiple=u32 500) -> ()  [unwired: 1 out]
        n61 = local read "V7045_U_ist"() -> (→"VOLTAGE":dbl)
        n62 = local read "V7045_I_ist"() -> (→"CURRENT":dbl)
        n63 = local read "PV_зазор"() -> (→"PV":dbl)
        n64 = local read "X140"() -> (w445:bool[])
        n65 = call "Метакон.vi"("Vak_in"="PT2") -> ("Vak_out_txt"=→"PT 2":string)  [unwired: 9 in, 1 out]
        n66 = call "Метакон.vi"("Vak_in"="PT3") -> ("Vak_out_txt"=→"PT 3":string)  [unwired: 9 in, 1 out]
        n67 = call "Метакон.vi"("Vak_in"="PT1") -> ("Vak_out_txt"=→"PT 1":string)  [unwired: 9 in, 1 out]
        n68 = Format Date/Time String(seconds (now)=w483) -> (date/time string=→"текущее время":string)  [unwired: 2 in]
        n69 = Number To Fractional String(number="Т1", precision (6)=w394) -> (F-format string=→"ПОДШ. 1.1":string)  [unwired: 2 in]
        n70 = Number To Fractional String(number="Т2", precision (6)=w394) -> (F-format string=→"ПОДШ. 1.2":string)  [unwired: 2 in]
        n71 = Number To Fractional String(number="Т3", precision (6)=w394) -> (F-format string=→"ПОДШ. 2.1":string)  [unwired: 2 in]
        n72 = Number To Fractional String(number="Т4", precision (6)=w394) -> (F-format string=→"ПОДШ. 2.2":string)  [unwired: 2 in]
        n73 = Number To Fractional String(number="Т5", precision (6)=w394) -> (F-format string=→"ТЕМП РОЛИК":string)  [unwired: 2 in]
        n74 = Number To Fractional String(number="Т6", precision (6)=w394) -> (F-format string=→"ТЕМП КАМЕРА":string)  [unwired: 2 in]
        n75 = call "presure PA.vi"("Volte"="PT3 2") -> ("presure String 2"=→"PT 4":string)  [unwired: 7 in, 3 out]
        n76 = Number To Boolean Array(number="x340") -> (Boolean array=→"X340":bool[])
        n77 = Number To Boolean Array(number="x200") -> (Boolean array=→"X200":bool[])
        n78 = Number To Boolean Array(number="x400") -> (Boolean array=→"X400":bool[])
        n79 = Number To Boolean Array(number="y120") -> (Boolean array=→"Y120":bool[])
        n80 = Number To Boolean Array(number="x140") -> (Boolean array=→"X140":bool[])
        n81 = Number To Boolean Array(number="x300") -> (Boolean array=→"X300":bool[])
        n82 = Number To Boolean Array(number="x240") -> (Boolean array=→"X240":bool[])
        n83 = Number To Boolean Array(number="x100") -> (Boolean array=→"X100":bool[])
        n84 = Number To Boolean Array(number="y60") -> (Boolean array=→"Y60":bool[])
        n85 = local read "V вращ. бараб"() -> (w510:string)
        n86 = local read "V барабаны 2"() -> (→"PULLEYS":dbl)
        n87 = Index Array(array=w551, index #1=2, index #2=5) -> ()  [unwired: 2 out]
        n88 = Number To Fractional String(number="PE3", precision (6)=i16 2) -> (F-format string=→"PE3" →"P camera (bar)":string)  [unwired: 2 in]
        n89 = Number To Fractional String(number="PE1", precision (6)=i16 2) -> (F-format string=→"PE1" →"P plasmatron (bar)":string)  [unwired: 2 in]
        n90 = Number To Fractional String(number="PE2", precision (6)=i16 1) -> (F-format string=→"PE2":string)  [unwired: 2 in]
        n91 = local read "Диаметр заг."() -> (w402:string)
        n92 = Index Array(array=w545, index #1=10, index #2=11, index #3=12) -> (element #1=w539:bool, element #2=w538:bool, element #3=w537:bool)
        n93 = Index Array(array=w473, index #1=27, index #2=29, index #3=30) -> (element #1=w477:bool, element #2=w480:bool, element #3=w481:bool)
        n94 = Index Array(array=w544, index #1=23, index #2=24, index #3=25, index #4=26) -> (element #1=w533:bool, element #2=w532:bool, element #3=w531:bool, element #4=w530:bool)
        n95 = Index Array(array=w625, index #1=16, index #2=18, index #3=19, index #4=20, index #5=21, index #6=24, index #7=25, index #8=28, index #9=29) -> (element #6=→"ролик_прижат":bool, element #7=→"ролик_отжат":bool, element #8=→"УГ_открыт":bool, element #9=→"УГ_закрыт":bool)  [unwired: 5 out]
        n96 = local read "U_ist"() -> (w505:string)
        n97 = To Long Integer(number="Скорость пп 2") -> (32bit integer=w399:i32)
        n98 = To Long Integer(number="Скорость пп") -> (32bit integer=w375:i32)
        n99 = Index Array(array=w606, index #1=1, index #2=6, index #3=7, index #4=27, index #5=14, index #6=13, index #7=21, index #8=22, index #9=23, index #10=24, index #11=25, index #12=19) -> ()  [unwired: 12 out]
        n100 = Index Array(array=w410, index #1=2, index #2=5, index #3=8, index #4=12, index #5=11, index #6=17, index #7=16, index #8=21, index #9=20, index #10=25, index #11=24, index #12=29, index #13=28) -> (element #1=w412:bool, element #2=w416:bool, element #3=w417:bool, element #4=w421:bool, element #5=w422:bool, element #6=w429:bool, element #7=w430:bool, element #8=w437:bool, element #9=w438:bool, element #10=w439:bool, element #11=w440:bool, element #12=w443:bool, element #13=w444:bool)
        n101 = Number To Fractional String(number="M_PLasmatron", precision (6)=i16 1) -> (F-format string=→"voto plasmatron":string)  [unwired: 2 in]
        n102 = Index Array(array=w590, index #1=16, index #2=17, index #3=18, index #4=19, index #5=20, index #6=9, index #7=12, index #8=13, index #9=16, index #10=17, index #11=18, index #12=19, index #13=21, index #14=22, index #15=23, index #16=27, index #17=28, index #18=29) -> (element #1=→"Air":bool, element #2=→"Air 4":bool, element #3=→"Water-1":bool, element #4=→"Water-2":bool)  [unwired: 14 out]
        n103 = Index Array(array=w565, index #1=0, index #2=1, index #3=8, index #4=9, index #5=12, index #6=13, index #7=20, index #8=21, index #9=22, index #10=23, index #11=24, index #12=25, index #13=26, index #14=27, index #15=28, index #16=29, index #17=30, index #18=31) -> (element #7=w564:bool, element #8=w563:bool, element #9=w562:bool, element #10=w561:bool, element #11=w560:bool, element #12=w559:bool, element #13=w558:bool, element #14=w557:bool, element #15=w556:bool, element #16=w555:bool, element #17=w554:bool)  [unwired: 7 out]
        n104 = Index Array(array=w445, index #1=4, index #2=5, index #3=6, index #4=9, index #5=8, index #6=11, index #7=10) -> (element #1=w456:bool, element #2=w457:bool, element #3=w458:bool, element #4=w461:bool, element #5=w462:bool, element #6=w470:bool, element #7=w469:bool)
        n105 = call "Индекс картинки.vi"("off"=w481, "on"=w480) -> ("index_image"=→"VP6":u16)  [unwired: 9 in]
        n106 = Decimal String To Number(string=w505) -> (number=w504:i32)  [unwired: 2 in, 1 out]
        n107 = Decimal String To Number(string=w510) -> (number=w509:i32)  [unwired: 2 in, 1 out]
        n108 = Boolean To (0,1)(Boolean=w539) -> (0, 1=→"EV1":i16)
        n109 = Boolean To (0,1)(Boolean=w538) -> (0, 1=→"EV2":i16)
        n110 = Boolean To (0,1)(Boolean=w533) -> (0, 1=→"CO1":i16)
        n111 = Boolean To (0,1)(Boolean=w532) -> (0, 1=→"CO2":i16)
        n112 = Boolean To (0,1)(Boolean=w531) -> (0, 1=→"CO3":i16)
        n113 = Boolean To (0,1)(Boolean=w530) -> (0, 1=→"P1":i16)
        n114 = Decimal String To Number(string=w402) -> (number=w365:i32)  [unwired: 2 in, 1 out]
        n115 = Boolean To (0,1)(Boolean=w477) -> (0, 1=→"NL 2":i16)
        n116 = Number To Decimal String(number=w399) -> (decimal integer string=w401:string)  [unwired: 1 in]
        n117 = Number To Decimal String(number=w375) -> (decimal integer string=w376:string)  [unwired: 1 in]
        n118 = Boolean To (0,1)(Boolean=w537) -> (0, 1=→"EV3.2" →"EV3.3" →"EV3.1":i16)
        n119 = Number To Fractional String(number="V барабаны задание", precision (6)=i16 0) -> (F-format string=→"V задания":string)  [unwired: 2 in]
        n120 = Multiply(x="ЗАДАНИЕ ТОКА", y=1.638) -> (x*y=w379:dbl)
        n121 = local read "Boolean"() -> (w355:bool)
        n122 = call "Индекс картинки.vi"("off"=w422, "on"=w421) -> ("index_image"=→"VP1":u16)  [unwired: 9 in]
        n123 = call "Индекс картинки.vi"("off"=w430, "on"=w429) -> ("index_image"=→"VP2":u16)  [unwired: 9 in]
        n124 = call "Индекс картинки.vi"("off"=w438, "on"=w437) -> ("index_image"=→"VP3":u16)  [unwired: 9 in]
        n125 = call "Индекс картинки.vi"("off"=w440, "on"=w439) -> ("index_image"=→"VP4":u16)  [unwired: 9 in]
        n126 = call "Индекс картинки.vi"("off"=w444, "on"=w443) -> ("index_image"=→"VP5":u16)  [unwired: 9 in]
        n127 = call "Индекс картинки.vi"("off"=w462, "on"=w461) -> ("index_image"=→"PD1":u16)  [unwired: 9 in]
        n128 = call "Индекс картинки.vi"("off"=w470, "on"=w469) -> ("index_image"=→"PD2":u16)  [unwired: 9 in]
        n129 = local write "Скорость ПП 2"(w401) -> ()
        n130 = local write "Скорость ПП"(w376) -> ()
        n131 = Boolean To (0,1)(Boolean=w412) -> (0, 1=→"NL":i16)
        n132 = Boolean To (0,1)(Boolean=w417) -> (0, 1=→"NB":i16)
        n133 = Boolean To (0,1)(Boolean=w416) -> (0, 1=→"NZ":i16)
        n134 = Boolean To (0,1)(Boolean=w458) -> (0, 1=→"PT3":i16)
        n135 = Boolean To (0,1)(Boolean=w456) -> (0, 1=→"PT1":i16)
        n136 = Boolean To (0,1)(Boolean=w457) -> (0, 1=→"PT2":i16)
        n137 = Equal?(x=w365, y=0) -> (x = y?=w368:bool)
        n138 = Greater Or Equal?(x=w504, y=20) -> (x >= y?=w502:bool)
        n139 = Greater Or Equal?(x=w509, y=500) -> (x >= y?=w507:bool)
        n140 = Build Array(w564, w563, w562, w561, w560, w559, w558, w557, w556, w555, w554) -> (w518:bool[])
        n141 = property on="Arhive" class="Bool"() -> ("DisabledEnum"=w353:T6)  [unwired: 2 in, 2 out]
        n142 = And(x=w502, y=w507) -> (x .and. y?=w506:bool)
        n143 = To Long Integer(number=w379) -> (32bit integer=w380:i32)
        n144 = local write "Запись отчета"(w506) -> ()
        n145 = event shown="[0] Timeout" {
          selector: _ -> [_]
          dyn-events: _ -> [_]
          timeout: _ -> [_]
          event Timeout {
            n146 = event-data() -> ()  [unwired: 1 in, 3 out]
          }
        }
        n147 = call "1.1 индикар полки.vi"("appended array"=w518) -> ("текущее положение"=→"ИНдикатор положения полки":string)  [unwired: 10 in]
        n148 = Number To Decimal String(number=w380) -> (decimal integer string=w381:string)  [unwired: 1 in]
        n149 = Not Equal?(x=w353, y=T6."Disabled and Grayed Out" ("Disabled")) -> (x != y?=w357:bool)
        n150 = Not Equal?(x=w353, y=T6."Enabled") -> (x != y?=w351:bool)
        n151 = case shown="False" w368 {
          tunnel: w365 -> [w628 _]
          tunnel: [w628 210] -> w364
          frame False {
          }
          frame True {
          }
        }
        n152 = And(x=w355, y=w357) -> (x .and. y?=w358:bool)
        n153 = case shown="True" w358 {
          frame False {
          }
          frame True {
            n154 = property on="Arhive" class="Bool"("DisabledEnum"=T6."Disabled and Grayed Out" ("Disabled")) -> ()  [unwired: 2 in, 2 out]
          }
        }
        n155 = Not(x=w355) -> (.not. x?=w354:bool)
        n156 = And(x=w354, y=w351) -> (x .and. y?=w350:bool)
        n157 = local write "задание тока А"(w381) -> ()
        n158 = case shown="True" w350 {
          frame False {
          }
          frame True {
            n159 = property on="Arhive" class="Bool"("DisabledEnum"=T6."Enabled" ("Disabled")) -> ()  [unwired: 2 in, 2 out]
          }
        }
        n160 = Divide(x=210.0, y=w364) -> (x/y=w362:dbl)
        n161 = Number To Decimal String(number="Position (mm)") -> (decimal integer string=→"String":string)  [unwired: 1 in]
        n162 = Multiply(x=9180, y=w362) -> (x*y=w360:dbl)
        n163 = Number To Fractional String(number=w360, precision (6)=i16 0) -> (F-format string=→"max Speed":string)  [unwired: 2 in]
        n164 = Multiply(x="V барабаны", y=w362) -> (x*y=w406:dbl)
        n165 = To Long Integer(number=w406) -> (32bit integer=w367:i32)
        "V барабаны 2" <- w367
        n166 = Number To Fractional String(number=w367, precision (6)=i16 0) -> (F-format string=→"V вращ. бараб":string)  [unwired: 2 in]
      }
      n167 = while {
        stop <- FALSE stop-if-true
        n168 = event shown="[0] \"Выход\": Value Change" {
          selector: _ -> [_ _ _ _ _ _ _ _ _ _ _ _ _ _ _ _ _ _ _ _ _ _ _ _ _ _ _ _]
          dyn-events: _ -> [_ _ _ _ _ _ _ _ _ _ _ _ _ _ _ _ _ _ _ _ _ _ _ _ _ _ _ _]
          timeout: _ -> [_ _ _ _ _ _ _ _ _ _ _ _ _ _ _ _ _ _ _ _ _ _ _ _ _ _ _ _]
          event "Выход": Value Change {
            n169 = event-data() -> ()  [unwired: 1 in, 5 out]
            n170 = Stop(stop? (T)="Выход") -> ()
          }
          event "Arhive": Value Change {
            n171 = event-data() -> ()  [unwired: 1 in, 5 out]
            n172 = call "1.3.форма базы отчетов.vi"() -> ()  [unwired: 12 in]
          }
          event "Сохранить настройки": Value Change {
            w147 = i16 0 ("precision (6)")
            n173 = event-data() -> ()  [unwired: 1 in, 5 out]
            n174 = local read "PARAMETERS VIDEO"() -> (w187:T3)
            n175 = local read "Индикатор камеры 2"() -> (w170:bool)
            n176 = local read "Индикатор камеры"() -> (w197:bool)
            n177 = local read "BINAR LEVEL"() -> (w173:cluster{"DOWN LEVEL":sgl, "UP LEVEL":sgl})
            n178 = local read "HOOK"() -> (w196:T2)
            n179 = Unbundle(w187) -> ("Contrast"=w186:i32, "Filter width"=w185:i32, "Steepness"=w184:i32, "Subsampling Ratio"=w183:u32, "Show Search Area"=w182:bool, "Show Search Lines"=w181:bool, "Show Edges Found"=w180:bool, "Show Result"=w179:bool)
            n180 = local read "WORK COLOR"() -> (w138:u32)
            n181 = local read "CALIBRATION"() -> (w174:u32)
            n182 = call <vilib>:"Application Directory.vi"() -> ("Application Directory"=w143:path)
            n183 = local read "SHEMA"() -> (w193:i32)
            n184 = local read "DELAY"() -> (w195:u32)
            n185 = Unbundle(w173) -> ("DOWN LEVEL"=w172:sgl, "UP LEVEL"=w171:sgl)
            n186 = Boolean To (0,1)(Boolean=w197) -> (0, 1=w194:i16)
            n187 = Boolean To (0,1)(Boolean=w182) -> (0, 1=w178:i16)
            n188 = Boolean To (0,1)(Boolean=w181) -> (0, 1=w177:i16)
            n189 = Boolean To (0,1)(Boolean=w180) -> (0, 1=w176:i16)
            n190 = Boolean To (0,1)(Boolean=w179) -> (0, 1=w175:i16)
            n191 = Boolean To (0,1)(Boolean=w170) -> (0, 1=w150:i16)
            n192 = Unbundle(w196) -> ("Left"=w192:i32, "Top"=w191:i32, "Right"=w190:i32, "Bottom"=w189:i32, "Rotation"=w188:dbl)
            n193 = Path To String(path=w143) -> (string=w142:string)
            n194 = Number To Fractional String(number=w178, precision (6)=w147) -> (F-format string=w157:string)  [unwired: 2 in]
            n195 = Number To Fractional String(number=w177, precision (6)=w147) -> (F-format string=w156:string)  [unwired: 2 in]
            n196 = Number To Fractional String(number=w176, precision (6)=w147) -> (F-format string=w155:string)  [unwired: 2 in]
            n197 = Number To Fractional String(number=w175, precision (6)=w147) -> (F-format string=w154:string)  [unwired: 2 in]
            n198 = Number To Fractional String(number=w195) -> (F-format string=w168:string)  [unwired: 3 in]
            n199 = Number To Fractional String(number=w193) -> (F-format string=w167:string)  [unwired: 3 in]
            n200 = Number To Fractional String(number=w192) -> (F-format string=w166:string)  [unwired: 3 in]
            n201 = Number To Fractional String(number=w191) -> (F-format string=w165:string)  [unwired: 3 in]
            n202 = Number To Fractional String(number=w190) -> (F-format string=w164:string)  [unwired: 3 in]
            n203 = Number To Fractional String(number=w189) -> (F-format string=w163:string)  [unwired: 3 in]
            n204 = Number To Fractional String(number=w188) -> (F-format string=w162:string)  [unwired: 3 in]
            n205 = Number To Fractional String(number=w186) -> (F-format string=w161:string)  [unwired: 3 in]
            n206 = Number To Fractional String(number=w185) -> (F-format string=w160:string)  [unwired: 3 in]
            n207 = Number To Fractional String(number=w184) -> (F-format string=w159:string)  [unwired: 3 in]
            n208 = Number To Fractional String(number=w183) -> (F-format string=w158:string)  [unwired: 3 in]
            n209 = Number To Fractional String(number=w174) -> (F-format string=w153:string)  [unwired: 3 in]
            n210 = Number To Fractional String(number=w172) -> (F-format string=w152:string)  [unwired: 3 in]
            n211 = Number To Fractional String(number=w171) -> (F-format string=w151:string)  [unwired: 3 in]
            n212 = Number To Fractional String(number=w194, precision (6)=i16 0) -> (F-format string=w169:string)  [unwired: 2 in]
            n213 = Number To Fractional String(number=w150, precision (6)=i16 0) -> (F-format string=w149:string)  [unwired: 2 in]
            n214 = Number To Fractional String(number=w138, precision (6)=i16 0) -> (F-format string=w136:string)  [unwired: 2 in]
            n215 = local read "CAM"() -> (w148:T1)
            n216 = Concatenate Strings(w142, "\\set_cam" ("string")) -> (w140:string)
            n217 = Build Array(w148, w169, w168, w167, w166, w165, w164, w163, w162, w161, w160, w159, w158, w157, w156, w155, w154, w153, w152, w151, w149, w136) -> (w144:T1[])
            n218 = String To Path(string=w140) -> (path=w139:path)
            n219 = call-poly <vilib>:"Write To Spreadsheet File.vi"("1D data"=w144, "file path (dialog if empty)"=w139) -> ()  [unwired: 6 in, 1 out]
          }
          event "V задания": Mouse Down {
            (unwired) "" ("ТЕКУЩЕЕ ЗНАЧЕНИЕ")
            n220 = event-data() -> ()  [unwired: 1 in, 7 out]
            n221 = local read "max Speed"() -> (w199:string)
            n222 = local read "V задания"() -> (w200:string)
            n223 = Decimal String To Number(string=w199) -> (number=w198:i32)  [unwired: 2 in, 1 out]
            n224 = call "NUMPAD1_9(ПРОГРАММА).vi"("МИНИМАЛЬНОЕ ЗНАЧЕНИЕ"=-1.0, "МАКСИМАЛЬНОЕ ЗНАЧЕНИЕ"=w198, "ДЛИННА СЛОВА"=i8 5, "ТЕКУЩЕЕ ЗНАЧЕНИЕ"=w200) -> ("НОВОЕ ЗНАЧЕНИЕ"=w202:string)  [unwired: 7 in]
            n225 = Fract/Exp String To Number(string=w202) -> (number=w201:dbl)  [unwired: 3 in, 1 out]
            n226 = DataSocket Write(8:errorcluster {"status"=FALSE, "code"=0, "source"=""} ("error in (no error)"), 9:500 ("ms timeout (0)"), 10:w201, 11:"opc://localhost/National Instruments.NIOPCServers/CNL_1.PLC1.PARAM_RASP.SP_S_MOVE" ("connection in")) -> ()  [unwired: 3 out]
          }
          event "Диаметр заг.": Mouse Down {
            n227 = event-data() -> ()  [unwired: 1 in, 7 out]
            n228 = local read "Диаметр заг."() -> (w208:string)
            n229 = call "NUMPAD1_9.vi"("МИНИМАЛЬНОЕ ЗНАЧЕНИЕ"=40.0, "МАКСИМАЛЬНОЕ ЗНАЧЕНИЕ"=90.0, "ДЛИННА СЛОВА"=i8 2, "ТЕКУЩЕЕ ЗНАЧЕНИЕ"=w208) -> ("НОВОЕ ЗНАЧЕНИЕ"=w213:string)  [unwired: 7 in]
            n230 = Fract/Exp String To Number(string=w213) -> (number=w212:dbl)  [unwired: 3 in, 1 out]
            n231 = Multiply(x=w212, y=10.0) -> (x*y=w210:dbl)
            n232 = To Word Integer(number=w210) -> (16bit integer=w209:i16)
            n233 = DataSocket Write(8:errorcluster {"status"=FALSE, "code"=0, "source"=""} ("error in (no error)"), 9:100 ("ms timeout (0)"), 10:w209, 11:"opc://localhost/National Instruments.NIOPCServers/CNL_1.PLC1.PARAM_RASP.D_ZAG") -> (0:w215:errorcluster)  [unwired: 2 out]
            n234 = Unbundle(w215) -> ()  [unwired: 3 out]
          }
          event "ГС -Открыть": Value Change {
            n235 = event-data() -> ()  [unwired: 1 in, 5 out]
            n236 = DataSocket Write(8:errorcluster {"status"=FALSE, "code"=0, "source"=""} ("error in (no error)"), 9:500 ("ms timeout (0)"), 10:TRUE, 11:"" ("connection in")) -> ()  [unwired: 3 out]
          }
          event "ГС - Закрыть": Value Change {
            n237 = event-data() -> ()  [unwired: 1 in, 5 out]
            n238 = DataSocket Write(8:errorcluster {"status"=FALSE, "code"=0, "source"=""} ("error in (no error)"), 9:500 ("ms timeout (0)"), 10:TRUE, 11:"" ("connection in")) -> ()  [unwired: 3 out]
          }
          event "Продол назад": Value Change {
            n239 = event-data() -> ()  [unwired: 1 in, 5 out]
            n240 = DataSocket Write(8:errorcluster {"status"=FALSE, "code"=0, "source"=""} ("error in (no error)"), 9:500 ("ms timeout (0)"), 10:TRUE, 11:"opc://localhost/National Instruments.NIOPCServers/CNL_1.PLC1.Makro.c601" ("connection in")) -> ()  [unwired: 3 out]
          }
          event "Продол впер": Value Change {
            n241 = event-data() -> ()  [unwired: 1 in, 5 out]
            n242 = local read "Порядковый номер"() -> (w236:string)
            n243 = Decimal String To Number(string=w236) -> (number=w235:i32)  [unwired: 2 in, 1 out]
            n244 = Increment(x=w235) -> (x+1=w234:i32)
            n245 = Number To Decimal String(number=w234) -> (decimal integer string=w233:string)  [unwired: 1 in]
            n246 = local write "Порядковый номер"(w233) -> ()
            n247 = DataSocket Write(8:errorcluster {"status"=FALSE, "code"=0, "source"=""} ("error in (no error)"), 9:500 ("ms timeout (0)"), 10:TRUE, 11:"opc://localhost/National Instruments.NIOPCServers/CNL_1.PLC1.Makro.c602" ("connection in")) -> ()  [unwired: 3 out]
          }
          event "ПОДАЧА ЗАГОТОВКИ": Value Change {
            n248 = event-data() -> ()  [unwired: 1 in, 5 out]
            n249 = DataSocket Write(8:errorcluster {"status"=FALSE, "code"=0, "source"=""} ("error in (no error)"), 9:250 ("ms timeout (0)"), 10:TRUE, 11:"opc://localhost/National Instruments.NIOPCServers/DL.DL260.Buttons.Заг-набар" ("connection in")) -> (0:w241:errorcluster)  [unwired: 2 out]
            n250 = Unbundle(w241) -> ()  [unwired: 3 out]
          }
          event "Автораспыление доплавить": Value Change {
            n251 = event-data() -> ()  [unwired: 1 in, 5 out]
          }
          event "Автораспыление начать": Value Change {
            n252 = event-data() -> ()  [unwired: 1 in, 5 out]
            n253 = DataSocket Write(8:errorcluster {"status"=FALSE, "code"=0, "source"=""} ("error in (no error)"), 9:250 ("ms timeout (0)"), 10:TRUE, 11:"opc://localhost/National Instruments.NIOPCServers/DL.DL260.Buttons.расплав-начать" ("connection in")) -> ()  [unwired: 3 out]
          }
          event "ПЛАЗМАТРОН В ИСХОДНОЕ": Value Change {
            n254 = event-data() -> ()  [unwired: 1 in, 5 out]
            n255 = DataSocket Write(8:errorcluster {"status"=FALSE, "code"=0, "source"=""} ("error in (no error)"), 9:500 ("ms timeout (0)"), 10:TRUE, 11:"opc://localhost/National Instruments.NIOPCServers/CNL_1.PLC1.Makro.c600" ("connection in")) -> ()  [unwired: 3 out]
          }
          event "Закончить автораспыление": Value Change {
            n256 = event-data() -> ()  [unwired: 1 in, 5 out]
            n257 = DataSocket Write(8:errorcluster {"status"=FALSE, "code"=0, "source"=""} ("error in (no error)"), 9:250 ("ms timeout (0)"), 10:TRUE, 11:"opc://localhost/National Instruments.NIOPCServers/DL.DL260.Buttons.расплав-закончить" ("connection in")) -> ()  [unwired: 3 out]
          }
          event "Скорость ПП": Mouse Down {
            n258 = event-data() -> ()  [unwired: 1 in, 7 out]
            n259 = call "NUMPAD1_9.vi"("МИНИМАЛЬНОЕ ЗНАЧЕНИЕ"=0.0, "МАКСИМАЛЬНОЕ ЗНАЧЕНИЕ"=601.0, "ДЛИННА СЛОВА"=i8 3, "ТЕКУЩЕЕ ЗНАЧЕНИЕ"="Скорость ПП") -> ("НОВОЕ ЗНАЧЕНИЕ"=w266:string)  [unwired: 7 in]
            n260 = Decimal String To Number(string=w266) -> (number=w258:i32)  [unwired: 2 in, 1 out]
            n261 = To Long Integer(number=w258) -> (32bit integer=w259:i32)
            n262 = DataSocket Write(8:errorcluster {"status"=FALSE, "code"=0, "source"=""} ("error in (no error)"), 9:250 ("ms timeout (0)"), 10:w259, 11:"opc://localhost/National Instruments.NIOPCServers/CNL_1.PLC1.PARAM_RASP.OUT_P_SAG_M" ("connection in")) -> ()  [unwired: 3 out]
            n263 = DataSocket Write(8:errorcluster {"status"=FALSE, "code"=0, "source"=""} ("error in (no error)"), 9:250 ("ms timeout (0)"), 10:w259, 11:"opc://localhost/National Instruments.NIOPCServers/CNL_1.PLC1.PARAM_RASP.4165" ("connection in")) -> ()  [unwired: 3 out]
          }
          event "Скорость ПП 2": Mouse Down {
            n264 = event-data() -> ()  [unwired: 1 in, 7 out]
            n265 = call "NUMPAD1_9.vi"("МИНИМАЛЬНОЕ ЗНАЧЕНИЕ"=0.0, "МАКСИМАЛЬНОЕ ЗНАЧЕНИЕ"=361.0, "ДЛИННА СЛОВА"=i8 3, "ТЕКУЩЕЕ ЗНАЧЕНИЕ"="Скорость ПП 2") -> ("НОВОЕ ЗНАЧЕНИЕ"=w280:string)  [unwired: 7 in]
            n266 = Decimal String To Number(string=w280) -> (number=w272:i32)  [unwired: 2 in, 1 out]
            n267 = To Long Integer(number=w272) -> (32bit integer=w273:i32)
            n268 = DataSocket Write(8:errorcluster {"status"=FALSE, "code"=0, "source"=""} ("error in (no error)"), 9:250 ("ms timeout (0)"), 10:w273, 11:"opc://localhost/National Instruments.NIOPCServers/CNL_1.PLC1.PARAM_RASP.SP_PR_PLAZM" ("connection in")) -> ()  [unwired: 3 out]
            n269 = DataSocket Write(8:errorcluster {"status"=FALSE, "code"=0, "source"=""} ("error in (no error)"), 9:250 ("ms timeout (0)"), 10:w273, 11:"opc://localhost/National Instruments.NIOPCServers/CNL_1.PLC1.PARAM_RASP.4166" ("connection in")) -> ()  [unwired: 3 out]
          }
          event "МАКСИМАЛЬНАЯ СКОРОСТЬ ПП К": Value Change {
            w284 = "opc://localhost/National Instruments.NIOPCServers/CNL_1.PLC1.PARAM_RASP.SP_PR_PLAZM"  # opc://localhost/National Instruments.NIOPCServers/CNL_1.PLC1.PARAM_RASP.SP_PR_PLAZM
            w288 = "opc://localhost/National Instruments.NIOPCServers/CNL_1.PLC1.PARAM_RASP.SP_PR_ZAG"  # opc://localhost/National Instruments.NIOPCServers/CNL_1.PLC1.PARAM_RASP.SP_PR_ZAG
            n270 = event-data() -> ()  [unwired: 1 in, 5 out]
            n271 = DataSocket Write(8:errorcluster {"status"=FALSE, "code"=0, "source"=""} ("error in (no error)"), 10:600, 11:w288) -> ()  [unwired: 1 in, 3 out]
            n272 = DataSocket Write(8:errorcluster {"status"=FALSE, "code"=0, "source"=""} ("error in (no error)"), 10:360, 11:w284) -> ()  [unwired: 1 in, 3 out]
          }
          event "задание тока А": Mouse Down {
            n273 = event-data() -> ()  [unwired: 1 in, 7 out]
            n274 = call "NUMPAD1_9.vi"("МИНИМАЛЬНОЕ ЗНАЧЕНИЕ"=0.0, "МАКСИМАЛЬНОЕ ЗНАЧЕНИЕ"=2500.0, "ДЛИННА СЛОВА"=i8 4, "ТЕКУЩЕЕ ЗНАЧЕНИЕ"="задание тока А") -> ("НОВОЕ ЗНАЧЕНИЕ"=w298:string)  [unwired: 7 in]
            n275 = Decimal String To Number(string=w298) -> (number=w297:i32)  [unwired: 2 in, 1 out]
            n276 = Multiply(x=w297, y=1.638) -> (x*y=w295:dbl)
            n277 = To Long Integer(number=w295) -> (32bit integer=w294:i32)
            n278 = DataSocket Write(8:errorcluster {"status"=FALSE, "code"=0, "source"=""} ("error in (no error)"), 9:250 ("ms timeout (0)"), 10:w294, 11:"opc://localhost/National Instruments.NIOPCServers/DL.DL260.Vmem.ист-задание" ("connection in")) -> ()  [unwired: 3 out]
          }
          event "Улавливатель закрыть": Value Change {
            n279 = event-data() -> ()  [unwired: 1 in, 5 out]
          }
          event "Улавливатель открыть": Value Change {
            n280 = event-data() -> ()  [unwired: 1 in, 5 out]
          }
          event "Ролик прижать": Value Change {
            n281 = event-data() -> ()  [unwired: 1 in, 5 out]
            n282 = DataSocket Write(8:errorcluster {"status"=FALSE, "code"=0, "source"=""} ("error in (no error)"), 9:500 ("ms timeout (0)"), 10:TRUE, 11:"opc://localhost/National Instruments.NIOPCServers/DL.DL260.Buttons.Рол-прижать" ("connection in")) -> ()  [unwired: 3 out]
          }
          event "Ролик отжать": Value Change {
            n283 = event-data() -> ()  [unwired: 1 in, 5 out]
            n284 = DataSocket Write(8:errorcluster {"status"=FALSE, "code"=0, "source"=""} ("error in (no error)"), 9:500 ("ms timeout (0)"), 10:TRUE, 11:"opc://localhost/National Instruments.NIOPCServers/DL.DL260.Buttons.Рол-отжать" ("connection in")) -> ()  [unwired: 3 out]
          }
          event "откачать рабочий вакуум": Value Change {
            n285 = event-data() -> ()  [unwired: 1 in, 5 out]
            n286 = property on="откачать рабочий вакуум" class="Bool"() -> ("BoolText.Text"=w315:string)  [unwired: 2 in, 2 out]
            n287 = call "Диалог_на_Макро.vi"("СОСТОЯНИЕ"="mac 2", "String"=w315) -> ("ВЫХОД"=w311:bool)  [unwired: 9 in]
            n288 = DataSocket Write(9:500 ("ms timeout (0)"), 10:w311, 11:"opc://localhost/National Instruments.NIOPCServers/CNL_1.PLC1.Makro.c200" ("connection in")) -> (0:w314:errorcluster)  [unwired: 1 in, 2 out]
            n289 = Unbundle(w314) -> ()  [unwired: 3 out]
          }
          event "forvacuum": Value Change {
            n290 = event-data() -> ()  [unwired: 1 in, 5 out]
            n291 = property on="forvacuum" class="Bool"() -> ("BoolText.Text"=w316:string)  [unwired: 2 in, 2 out]
            n292 = call "Диалог_на_Макро.vi"("СОСТОЯНИЕ"="forvakuum led", "String"=w316) -> ("ВЫХОД"=w321:bool)  [unwired: 9 in]
            n293 = DataSocket Write(9:500 ("ms timeout (0)"), 10:w321, 11:"opc://localhost/National Instruments.NIOPCServers/CNL_1.PLC1.Makro.c251" ("connection in")) -> (0:w318:errorcluster)  [unwired: 1 in, 2 out]
            n294 = Unbundle(w318) -> ()  [unwired: 3 out]
          }
          event "ND HEAT BUT": Value Change {
            n295 = event-data() -> ()  [unwired: 1 in, 5 out]
            n296 = property on="ND HEAT BUT" class="Bool"() -> ("BoolText.Text"=w322:string)  [unwired: 2 in, 2 out]
            n297 = call "Диалог_на_Макро.vi"("СОСТОЯНИЕ"="ND HEAT LED", "String"=w322) -> ("ВЫХОД"=w327:bool)  [unwired: 9 in]
            n298 = DataSocket Write(9:500 ("ms timeout (0)"), 10:w327, 11:"opc://localhost/National Instruments.NIOPCServers/CNL_1.PLC1.Makro.c250" ("connection in")) -> (0:w324:errorcluster)  [unwired: 1 in, 2 out]
            n299 = Unbundle(w324) -> ()  [unwired: 3 out]
          }
          event "откачка стоп": Value Change {
            n300 = event-data() -> ()  [unwired: 1 in, 5 out]
            n301 = property on="откачка стоп" class="Bool"() -> ("BoolText.Text"=w328:string)  [unwired: 2 in, 2 out]
            n302 = call "Диалог_на_Макро.vi"("СОСТОЯНИЕ"="mac3", "String"=w328) -> ("ВЫХОД"=w330:bool)  [unwired: 9 in]
            n303 = DataSocket Write(9:500 ("ms timeout (0)"), 10:w330, 11:"opc://localhost/National Instruments.NIOPCServers/CNL_1.PLC1.Makro.c201" ("connection in")) -> (0:w333:errorcluster)  [unwired: 1 in, 2 out]
            n304 = Unbundle(w333) -> ()  [unwired: 3 out]
          }
          event "напустить аргон": Value Change {
            n305 = event-data() -> ()  [unwired: 1 in, 5 out]
            n306 = property on="напустить аргон" class="Bool"() -> ("BoolText.Text"=w339:string)  [unwired: 2 in, 2 out]
            n307 = call "Диалог_на_Макро.vi"("СОСТОЯНИЕ"="mac 4", "String"=w339) -> ("ВЫХОД"=w334:bool)  [unwired: 9 in]
            n308 = DataSocket Write(9:500 ("ms timeout (0)"), 10:w334, 11:"opc://localhost/National Instruments.NIOPCServers/CNL_1.PLC1.Makro.napusk" ("connection in")) -> (0:w337:errorcluster)  [unwired: 1 in, 2 out]
            n309 = Unbundle(w337) -> ()  [unwired: 3 out]
          }
          event "ЗУ-вверх": Value Change {
            n310 = event-data() -> ()  [unwired: 1 in, 5 out]
            n311 = DataSocket Write(8:errorcluster {"status"=FALSE, "code"=0, "source"=""} ("error in (no error)"), 9:500 ("ms timeout (0)"), 10:TRUE, 11:"opc://localhost/National Instruments.NIOPCServers/CNL_1.PLC1.Makro.s226" ("connection in")) -> ()  [unwired: 3 out]
          }
        }
        n312 = Wait Until Next ms Multiple(millisecond multiple=u32 500) -> ()  [unwired: 1 out]
      }
      n313 = while {
        stop <- FALSE stop-if-true
        n314 = Get Date/Time In Seconds() -> (seconds since 1Jan1904=w104:timestamp)
        n315 = Wait (ms)(milliseconds to wait=u32 500) -> ()  [unwired: 1 out]
        n316 = Format Date/Time String(seconds (now)=w104) -> (date/time string=w98:string)  [unwired: 2 in]
        n317 = Greater?(x="Ошибка 2", y=i16 0) -> (0:w100:bool)
        n318 = case shown="True" w100 {
          tunnel: "Ошибка 2" -> [_ w117]
          tunnel: w98 -> [_ w114]
          frame False {
          }
          frame True {
            w106 = "\r"
            w116 = "\t"
            n319 = call "описание ошибки.vi"("Numeric"=w117) -> ("String 2"=w107:string, "String"=w111:string)  [unwired: 9 in]
            n320 = local write "Ошибка 2"(i16 0 ("Ошибка 2")) -> ()
            n321 = Number To Decimal String(number=w117) -> (decimal integer string=w112:string)  [unwired: 1 in]
            n322 = call "путь для общего отчета.vi"() -> ("path_out 2"=w118:string)  [unwired: 11 in]
            n323 = Concatenate Strings(w114, w116, w112, w116, w111, "   " ("string"), w107, "\n") -> (w119:string)
            n324 = Concatenate Strings("Data: " ("string"), w114, w106, "Numer: " ("string"), w112, w106, w111, w106, w107) -> (w110:string)
            n325 = Concatenate Strings(w118, "errors.txt") -> (w130:string)
            n326 = call "2.6. форма ошибки.vi"("Описание ошибки"=w110) -> ()  [unwired: 11 in]
            n327 = String To Path(string=w130) -> (path=w132:path)
            n328 = Open/Create/Replace File(file path (use dialog)=w132, error in=errorcluster {"status"=FALSE, "code"=0, "source"=""}, operation (0:open)=T5."open or create") -> (refnum out=w125:refnum<file>, error out=w127:errorcluster)  [unwired: 3 in, 1 out]
            n329 = Set File Position(refnum=w125, from (0:start)=enum16{"start", "end", "current"}."end", error in=w127) -> (refnum out=w123:refnum<file>, error out=w124:errorcluster)  [unwired: 1 in]
            n330 = Write to Text File(file (use dialog)=w123, text=w119, error in=w124) -> (refnum out=w122:refnum<file>, error out=w121:errorcluster)  [unwired: 1 in, 1 out]
            n331 = Close File(refnum=w122, error in=w121) -> (error out=w120:errorcluster)  [unwired: 1 out]
            n332 = Unbundle(w120) -> ()  [unwired: 3 out]
          }
        }
      }
    }
  }
  n333 = while {
    stop <- "stop 2" stop-if-true
    n334 = Wait Until Next ms Multiple(millisecond multiple=u32 250) -> ()  [unwired: 1 out]
    n335 = event shown="[2] \"Порядковый номер\": Mouse Down" {
      selector: _ -> [_ _ _ _ _ _ _ _ _ _ _]
      dyn-events: _ -> [_ _ _ _ _ _ _ _ _ _ _]
      timeout: 250 -> [_ _ _ _ _ _ _ _ _ _ _]
      event Timeout {
        n336 = event-data() -> ()  [unwired: 1 in, 2 out]
        n337 = local read "D, заготовки"() -> (w649:i16)
        n338 = Number To Decimal String(number="max out") -> (decimal integer string=→"Максимальная подача (мм/мин)2":string)  [unwired: 1 in]
        n339 = Number To Decimal String(number="out") -> (decimal integer string=→"Actual speed\n(mm/min)":string)  [unwired: 1 in]
        n340 = Number To Fractional String(number="SP_зазор", precision (6)=i16 1) -> (F-format string=→"SP (mm)":string)  [unwired: 2 in]
        n341 = Number To Fractional String(number="V7045_I_ist", precision (6)=i16 0) -> (F-format string=→"I_ist":string)  [unwired: 2 in]
        n342 = Number To Fractional String(number="PV_зазор", precision (6)=i16 1) -> (F-format string=→"PV(mm)":string)  [unwired: 2 in]
        n343 = Number To Decimal String(number="V7045_U_ist") -> (decimal integer string=→"U_ist":string)  [unwired: 1 in]
        n344 = Divide(x=w649, y=i16 10) -> (x/y=w647:dbl)
        n345 = Number To Decimal String(number="v4065_cкорость подачи") -> (decimal integer string=→"LONGITUDINAL SPEED":string)  [unwired: 1 in]
        n346 = Number To Decimal String(number=w647) -> (decimal integer string=→"Диаметр заг.":string)  [unwired: 1 in]
        n347 = Number To Decimal String(number="v4066_cкорость подачи плазматрона") -> (decimal integer string=→"PLASMATRON SPEED":string)  [unwired: 1 in]
      }
      event "ПЛАЗМАТРОН В ИСХОДНОЕ 2": Value Change {
        w689 = "D:\\img\\"
        w678 = enum32{"File", "Clipboard"}."File" ("Target")
        w679 = enum32{"BMP", "EPS", "EMF", "PICT"}."BMP" ("File Type")
        n348 = event-data() -> ()  [unwired: 1 in, 4 out]
        n349 = Get Date/Time In Seconds() -> (seconds since 1Jan1904=w668:timestamp)
        n350 = Get Date/Time String(seconds (now)=w668) -> ()  [unwired: 2 in, 2 out]
        n351 = Format Date/Time String(time format string (%c)="%H_%M_%S", seconds (now)=w668) -> (date/time string=w664:string)  [unwired: 1 in]
        n352 = Concatenate Strings("VOLTAGE-", w664) -> (w662:string)
        n353 = Concatenate Strings("CURRENT", w664) -> (w660:string)
        n354 = Concatenate Strings("PV-", w664) -> (w666:string)
        n355 = Concatenate Strings("FEED-", w664) -> (w656:string)
        n356 = Concatenate Strings(w689, w660) -> (w686:string)
        n357 = Concatenate Strings(w689, w662) -> (w688:string)
        n358 = Concatenate Strings("PULLEYS", w664) -> (w658:string)
        n359 = Concatenate Strings(w689, w666) -> (w687:string)
        n360 = String To Path(string=w686) -> (path=w682:path)
        n361 = String To Path(string=w688) -> (path=w669:path)
        n362 = Concatenate Strings(w689, w656) -> (w684:string)
        n363 = Concatenate Strings(w689, w658) -> (w685:string)
        n364 = String To Path(string=w687) -> (path=w683:path)
        n365 = String To Path(string=w684) -> (path=w680:path)
        n366 = String To Path(string=w685) -> (path=w681:path)
        n367 = invoke on="LONGITUDINAL FEED" class="WFChart (strict)" method="Export Image"("FileType"=w679, "Target"=w678, "Path"=w680) -> (error out=w673:errorcluster)  [unwired: 5 in, 7 out]
        n368 = invoke on="VOLTAGE" class="WFChart (strict)" method="Export Image"(error in=errorcluster {"status"=FALSE, "code"=0, "source"=""} ("error in (no error)"), "FileType"=w679, "Target"=w678, "Path"=w669, "HideGrid"=FALSE ("Hide Grid"), "Overwrite"=FALSE ("Always Overwrite")) -> (error out=w677:errorcluster)  [unwired: 2 in, 7 out]
        n369 = invoke on="PV" class="WFChart (strict)" method="Export Image"("FileType"=w679, "Target"=w678, "Path"=w683) -> (error out=w676:errorcluster)  [unwired: 5 in, 7 out]
        n370 = invoke on="CURRENT" class="WFChart (strict)" method="Export Image"("FileType"=w679, "Target"=w678, "Path"=w682) -> (error out=w675:errorcluster)  [unwired: 5 in, 7 out]
        n371 = invoke on="PULLEYS" class="WFChart (strict)" method="Export Image"("FileType"=w679, "Target"=w678, "Path"=w681) -> (error out=w674:errorcluster)  [unwired: 5 in, 7 out]
        n372 = Unbundle(w676) -> ()  [unwired: 3 out]
        n373 = Unbundle(w675) -> ()  [unwired: 3 out]
        n374 = Unbundle(w677) -> ()  [unwired: 3 out]
        n375 = Unbundle(w673) -> ()  [unwired: 3 out]
        n376 = Unbundle(w674) -> ()  [unwired: 3 out]
      }
      event "Порядковый номер": Mouse Down {
        n377 = event-data() -> ()  [unwired: 1 in, 4 out]
        n378 = local read "Порядковый номер"() -> (w694:string)
        n379 = call "NUMPAD1_9.vi"("МИНИМАЛЬНОЕ ЗНАЧЕНИЕ"=-1.0, "МАКСИМАЛЬНОЕ ЗНАЧЕНИЕ"=100.0, "ДЛИННА СЛОВА"=i8 2, "ТЕКУЩЕЕ ЗНАЧЕНИЕ"=w694) -> ("НОВОЕ ЗНАЧЕНИЕ"=w690:string)  [unwired: 7 in]
        n380 = local write "Порядковый номер"(w690) -> ()
      }
      event "PLASMATRON SPEED": Mouse Down {
        n381 = event-data() -> ()  [unwired: 1 in, 3 out]
        n382 = local read "PLASMATRON SPEED"() -> (w695:string)
        n383 = call "NUMPAD1_9.vi"("МИНИМАЛЬНОЕ ЗНАЧЕНИЕ"=0.0, "МАКСИМАЛЬНОЕ ЗНАЧЕНИЕ"=501.0, "ДЛИННА СЛОВА"=i8 3, "ТЕКУЩЕЕ ЗНАЧЕНИЕ"=w695) -> ("НОВОЕ ЗНАЧЕНИЕ"=w697:string)  [unwired: 7 in]
        n384 = Decimal String To Number(string=w697) -> (number=w700:i32)  [unwired: 2 in, 1 out]
        n385 = DataSocket Write(8:errorcluster {"status"=FALSE, "code"=0, "source"=""} ("error in (no error)"), 9:500 ("ms timeout (0)"), 10:w700, 11:"opc://localhost/National Instruments.NIOPCServers/CNL_1.PLC1.PARAM_RASP.SP_PR_PLAZM") -> (0:w703:errorcluster)  [unwired: 2 out]
        n386 = Unbundle(w703) -> ()  [unwired: 3 out]
      }
      event "LONGITUDINAL SPEED": Mouse Down {
        n387 = event-data() -> ()  [unwired: 1 in, 3 out]
        n388 = local read "LONGITUDINAL SPEED"() -> (w708:string)
        n389 = call "NUMPAD1_9.vi"("МИНИМАЛЬНОЕ ЗНАЧЕНИЕ"=0.0, "МАКСИМАЛЬНОЕ ЗНАЧЕНИЕ"=501.0, "ДЛИННА СЛОВА"=i8 3, "ТЕКУЩЕЕ ЗНАЧЕНИЕ"=w708) -> ("НОВОЕ ЗНАЧЕНИЕ"=w706:string)  [unwired: 7 in]
        n390 = Decimal String To Number(string=w706) -> (number=w710:i32)  [unwired: 2 in, 1 out]
        n391 = DataSocket Write(8:errorcluster {"status"=FALSE, "code"=0, "source"=""} ("error in (no error)"), 9:500 ("ms timeout (0)"), 10:w710, 11:"opc://localhost/National Instruments.NIOPCServers/CNL_1.PLC1.PARAM_RASP.OUT_P_SAG_M") -> (0:w713:errorcluster)  [unwired: 2 out]
        n392 = Unbundle(w713) -> ()  [unwired: 3 out]
      }
      event "Максимальная подача (мм/мин)2": Mouse Down {
        n393 = event-data() -> ()  [unwired: 1 in, 3 out]
        n394 = local read "Максимальная подача (мм/мин)2"() -> (w715:string)
        n395 = call "NUMPAD1_9.vi"("МИНИМАЛЬНОЕ ЗНАЧЕНИЕ"=0.1, "МАКСИМАЛЬНОЕ ЗНАЧЕНИЕ"=101.0, "ДЛИННА СЛОВА"=i8 3, "ТЕКУЩЕЕ ЗНАЧЕНИЕ"=w715) -> ("НОВОЕ ЗНАЧЕНИЕ"=w717:string)  [unwired: 7 in]
        n396 = Decimal String To Number(string=w717) -> (number=w716:i32)  [unwired: 2 in, 1 out]
        n397 = DataSocket Write(8:errorcluster {"status"=FALSE, "code"=0, "source"=""} ("error in (no error)"), 9:500 ("ms timeout (0)"), 10:w716, 11:"opc://localhost/National Instruments.NIOPCServers/CNL_1.PLC1.RID.MAX_OUT") -> (0:w723:errorcluster)  [unwired: 2 out]
        n398 = Unbundle(w723) -> ()  [unwired: 3 out]
      }
      event "Регулятор": Value Change {
        n399 = event-data() -> ()  [unwired: 1 in, 2 out]
        n400 = local read "Boolean"() -> (w726:bool)
        n401 = Not(x=w726) -> (.not. x?=w725:bool)
        n402 = DataSocket Write(8:errorcluster {"status"=FALSE, "code"=0, "source"=""} ("error in (no error)"), 9:500 ("ms timeout (0)"), 10:w725, 11:"opc://localhost/National Instruments.NIOPCServers/CNL_1.PLC1.RID.RID_RUN") -> (0:w729:errorcluster)  [unwired: 2 out]
        n403 = Unbundle(w729) -> ()  [unwired: 3 out]
      }
      event "взять зазор": Value Change {
        n404 = event-data() -> ()  [unwired: 1 in, 3 out]
        n405 = DataSocket Write(8:errorcluster {"status"=FALSE, "code"=0, "source"=""} ("error in (no error)"), 9:500 ("ms timeout (0)"), 10:TRUE, 11:"opc://localhost/National Instruments.NIOPCServers/CNL_1.PLC1.RID.PV_to_SP") -> (0:w733:errorcluster)  [unwired: 2 out]
        n406 = Unbundle(w733) -> ()  [unwired: 3 out]
      }
      event "SP (mm)": Mouse Down {
        n407 = event-data() -> ()  [unwired: 1 in, 2 out]
        n408 = local read "SP (mm)"() -> (w738:string)
        n409 = call "NUMPAD1_9(ПРОГРАММА).vi"("МИНИМАЛЬНОЕ ЗНАЧЕНИЕ"=0.09, "МАКСИМАЛЬНОЕ ЗНАЧЕНИЕ"=100.0, "ДЛИННА СЛОВА"=i8 4, "ТЕКУЩЕЕ ЗНАЧЕНИЕ"=w738) -> ("НОВОЕ ЗНАЧЕНИЕ"=w739:string)  [unwired: 7 in]
        n410 = Fract/Exp String To Number(string=w739) -> (number=w736:dbl)  [unwired: 3 in, 1 out]
        n411 = DataSocket Write(8:errorcluster {"status"=FALSE, "code"=0, "source"=""} ("error in (no error)"), 9:500 ("ms timeout (0)"), 10:w736, 11:"opc://localhost/National Instruments.NIOPCServers/CNL_1.PLC1.RID.SP_ZAZOR") -> (0:w744:errorcluster)  [unwired: 2 out]
        n412 = Unbundle(w744) -> ()  [unwired: 3 out]
      }
      event "Марка сплава": Mouse Down {
        n413 = event-data() -> ()  [unwired: 1 in, 4 out]
        n414 = local read "Марка сплава"() -> (w746:string)
        n415 = call "КЛАВИАТУРА ПОЛНАЯSMALL.vi"("ВХОД СТАРОЕ"=w746) -> ("ВЫХОД РЕЗУЛЬТАТ"=→"Марка сплава":string)  [unwired: 10 in]
      }
      event "откачка стоп 2": Value Change {
        n416 = event-data() -> ()  [unwired: 1 in, 4 out]
        n417 = call "8.1 форма проверки натекания.vi"() -> ()  [unwired: 1 in]
      }
    }
  }
  n418 = while {
    stop <- "stop 3" stop-if-true
    n419 = Wait (ms)(milliseconds to wait=u32 100) -> ()  [unwired: 1 out]
    n420 = local read "16bit integer"() -> (w749:i16)
    n421 = DataSocket Write(8:errorcluster {"status"=FALSE, "code"=0, "source"=""} ("error in (no error)"), 9:100 ("ms timeout (0)"), 10:w749, 11:"opc://localhost/National Instruments.NIOPCServers/CNL_1.PLC1.RID.PV_ZAZOR") -> (0:w750:errorcluster)  [unwired: 2 out]
    n422 = Unbundle(w750) -> ()  [unwired: 3 out]
  }
  n423 = while {
    stop <- FALSE stop-if-true
    n424 = flat-sequence {
      tunnel: [w770] -> w763
      tunnel: [w769] -> w757
      tunnel: [w768] -> w755
      tunnel: w763 -> [w781]
      tunnel: [w780] -> w762
      tunnel: [w775] -> w758
      tunnel: w757 -> [w775]
      tunnel: w755 -> [w773]
      tunnel: w762 -> [w789]
      tunnel: [w788] -> w760
      tunnel: [w787] -> w759
      tunnel: w758 -> [w787]
      tunnel: w760 -> [_]
      tunnel: w759 -> [_]
      frame #0 {
        "Record" <- FALSE ("Rec.")
      }
      frame #1 {
        n425 = while {
          stop <- "Запись отчета" stop-if-true
          n426 = Wait Until Next ms Multiple(millisecond multiple=u32 1000) -> ()  [unwired: 1 out]
        }
      }
      frame #2 {
        n427 = local read "Порядковый номер"() -> (w768:string)
        n428 = local write "Record"(TRUE ("Rec.")) -> ()
        n429 = call "1.1.путь каталога отчета цикла.vi"("bilet_numer"=w768) -> ("path_out"=w769:string)  [unwired: 10 in]
        n430 = Concatenate Strings(w769, "rasp.txt" ("string")) -> (w771:string)
        n431 = String To Path(string=w771) -> (path=w770:path)
      }
      frame #3 {
        n432 = local read "Марка сплава"() -> (w774:string)
        n433 = Get Date/Time In Seconds() -> (seconds since 1Jan1904=w777:timestamp)
        n434 = Format Date/Time String(seconds (now)=w777) -> (date/time string=w776:string)  [unwired: 2 in]
        n435 = Concatenate Strings(w776, "  WORK ", w774, " NUMBER - ", w773) -> ()  [unwired: 1 out]
        n436 = Open/Create/Replace File(file path (use dialog)=w781, error in=errorcluster {"status"=FALSE, "code"=0, "source"=""}, operation (0:open)=T5."open or create") -> (refnum out=w786:refnum<file>, error out=w785:errorcluster)  [unwired: 3 in, 1 out]
        n437 = Close File(refnum=w786, error in=w785) -> (path=w780:path, error out=w784:errorcluster)
        n438 = Unbundle(w784) -> ()  [unwired: 3 out]
        "Порядковый номер" <- w773
      }
      frame #4 {
        n439 = while {
          tunnel: w789 -> [w807]
          tunnel: [w801] -> w788
          stop <- w817 stop-if-true
          w804 = "\t"
          n440 = local read "Запись отчета"() -> (w800:bool)
          n441 = Wait Until Next ms Multiple(millisecond multiple=u32 1000) -> ()  [unwired: 1 out]
          n442 = local read "Порядковый номер"() -> (w802:string)
          n443 = local read "Actual speed\n(mm/min)"() -> (w796:string)
          n444 = local read "P plasmatron (bar)"() -> (w791:string)
          n445 = local read "V вращ. бараб"() -> (w797:string)
          n446 = local read "Марка сплава"() -> (w790:string)
          n447 = Get Date/Time In Seconds() -> (seconds since 1Jan1904=w799:timestamp)
          n448 = local read "Диаметр заг."() -> (w798:string)
          n449 = local read "P camera (bar)"() -> (w792:string)
          n450 = Format Date/Time String(seconds (now)=w799) -> (date/time string=w805:string)  [unwired: 2 in]
          n451 = Not(x=w800) -> (.not. x?=w817:bool)
          n452 = local read "PV(mm)"() -> (w793:string)
          n453 = local read "U_ist"() -> (w794:string)
          n454 = Open/Create/Replace File(file path (use dialog)=w807, error in=errorcluster {"status"=FALSE, "code"=0, "source"=""}) -> (refnum out=w816:refnum<file>, error out=w814:errorcluster)  [unwired: 4 in, 1 out]
          n455 = local read "I_ist"() -> (w795:string)
          n456 = Concatenate Strings(w805, w804, w798, w804, w797, w804, w796, w804, w795, w804, w794, w804, w793, w804, w792, w804, w791, w804, w790, w804, w802, "\r") -> (w806:string)
          n457 = Set File Position(refnum=w816, from (0:start)=enum16{"start", "end", "current"}."end", error in=w814) -> (refnum out=w813:refnum<file>, error out=w812:errorcluster)  [unwired: 1 in]
          n458 = Write to Text File(file (use dialog)=w813, text=w806, error in=w812) -> (refnum out=w811:refnum<file>, error out=w810:errorcluster)  [unwired: 1 in, 1 out]
          n459 = Close File(refnum=w811, error in=w810) -> (path=w801:path, error out=w809:errorcluster)
          n460 = Unbundle(w809) -> ()  [unwired: 3 out]
        }
      }
      frame #5 {
      }
    }
    n461 = Wait Until Next ms Multiple(millisecond multiple=u32 1000) -> ()  [unwired: 1 out]
  }
  n462 = local write "Порядковый номер"("0" ("Порядковый номер")) -> ()
  n463 = while {
    stop <- FALSE stop-if-true
    n464 = flat-sequence {
      tunnel: [w914] -> w821
      frame #0 {
        n465 = call <vilib>:"Application Directory.vi"() -> ("Application Directory"=w828:path)
        n466 = Path To String(path=w828) -> (string=w827:string)
        n467 = Concatenate Strings(w827, "\\set_cam" ("string")) -> (w825:string)
        n468 = String To Path(string=w825) -> (path=w822:path)
        n469 = Get File Size(file=w822) -> (0:w824:errorcluster)  [unwired: 1 in, 2 out]
        n470 = Unbundle By Name(w824) -> ("status"=w823:bool)
        n471 = case shown="False" w823 {
          tunnel: w822 -> [w901 _]
          frame False {
            n472 = call-poly <vilib>:"Read From Spreadsheet File.vi"("file path (dialog if empty)"=w901) -> ("first row"=w900:string[])  [unwired: 6 in, 4 out]
            n473 = Index Array(array=w900, index #1=0 ("index"), index #2=2 ("index"), index #3=3 ("index"), index #4=4 ("index"), index #5=5 ("index"), index #6=6 ("index"), index #7=7 ("index"), index #8=8 ("index"), index #9=9 ("index"), index #10=10 ("index"), index #11=11 ("index"), index #12=12 ("index"), index #13=13 ("index"), index #14=14 ("index"), index #15=15 ("index"), index #16=16 ("index"), index #17=17 ("index"), index #18=18 ("index"), index #19=19 ("index"), index #20=20 ("index"), index #21=21 ("index")) -> (element #1=w898:string, element #2=w896:string, element #3=w893:string, element #4=w885:string, element #5=w883:string, element #6=w881:string, element #7=w879:string, element #8=w877:string, element #9=w868:string, element #10=w866:string, element #11=w864:string, element #12=w862:string, element #13=w860:string, element #14=w858:string, element #15=w856:string, element #16=w854:string, element #17=w844:string, element #18=w839:string, element #19=w837:string, element #20=w833:string, element #21=w829:string)
            n474 = local write "CAM"(w898) -> ()
            n475 = Decimal String To Number(string=w896) -> (number=w895:i32)  [unwired: 2 in, 1 out]
            n476 = Decimal String To Number(string=w885) -> (number=w890:i32)  [unwired: 2 in, 1 out]
            n477 = Decimal String To Number(string=w883) -> (number=w889:i32)  [unwired: 2 in, 1 out]
            n478 = Decimal String To Number(string=w881) -> (number=w888:i32)  [unwired: 2 in, 1 out]
            n479 = Decimal String To Number(string=w879) -> (number=w887:i32)  [unwired: 2 in, 1 out]
            n480 = Fract/Exp String To Number(string=w877) -> (number=w876:dbl)  [unwired: 3 in, 1 out]
            n481 = Decimal String To Number(string=w893) -> (number=w892:i32)  [unwired: 2 in, 1 out]
            n482 = Decimal String To Number(string=w868) -> (number=w874:i32)  [unwired: 2 in, 1 out]
            n483 = Decimal String To Number(string=w866) -> (number=w873:i32)  [unwired: 2 in, 1 out]
            n484 = Decimal String To Number(string=w864) -> (number=w872:i32)  [unwired: 2 in, 1 out]
            n485 = Decimal String To Number(string=w862) -> (number=w871:i32)  [unwired: 2 in, 1 out]
            n486 = Decimal String To Number(string=w860) -> (number=w853:i32)  [unwired: 2 in, 1 out]
            n487 = Decimal String To Number(string=w858) -> (number=w851:i32)  [unwired: 2 in, 1 out]
            n488 = Decimal String To Number(string=w856) -> (number=w849:i32)  [unwired: 2 in, 1 out]
            n489 = Decimal String To Number(string=w854) -> (number=w847:i32)  [unwired: 2 in, 1 out]
            n490 = Decimal String To Number(string=w844) -> (number=w843:i32)  [unwired: 2 in, 1 out]
            n491 = Decimal String To Number(string=w839) -> (number=w838:i32)  [unwired: 2 in, 1 out]
            n492 = Decimal String To Number(string=w837) -> (number=w836:i32)  [unwired: 2 in, 1 out]
            n493 = Decimal String To Number(string=w833) -> (number=w835:i32)  [unwired: 2 in, 1 out]
            n494 = Decimal String To Number(string=w829) -> (number=w831:i32)  [unwired: 2 in, 1 out]
            n495 = local write "DELAY"(w895) -> ()
            n496 = local write "CALIBRATION"(w843) -> ()
            n497 = local write "SHEMA"(w892) -> ()
            n498 = local write "WORK COLOR"(w831) -> ()
            n499 = Bundle(w890, w889, w888, w887, w876) -> (w891:cluster{i32, i32, i32, i32, dbl})  [unwired: 1 in]
            n500 = To Unsigned Long Integer(number=w871) -> (unsigned 32bit integer=w870:u32)
            n501 = call "конвертюга.vi"("Numeric"=w853) -> ("Boolean"=w852:bool)  [unwired: 10 in]
            n502 = call "конвертюга.vi"("Numeric"=w851) -> ("Boolean"=w850:bool)  [unwired: 10 in]
            n503 = call "конвертюга.vi"("Numeric"=w849) -> ("Boolean"=w848:bool)  [unwired: 10 in]
            n504 = call "конвертюга.vi"("Numeric"=w847) -> ("Boolean"=w846:bool)  [unwired: 10 in]
            n505 = call "конвертюга.vi"("Numeric"=w835) -> ("Boolean"=w834:bool)  [unwired: 10 in]
            n506 = Bundle(w838, w836) -> (w842:cluster{i32, i32})  [unwired: 1 in]
            n507 = local write "HOOK"(w891) -> ()
            n508 = local write "BINAR LEVEL"(w842) -> ()
            n509 = local write "Blank Button"(w834) -> ()
            n510 = Bundle(w874, w873, w872, w870, "Boolean"=w852, "Boolean"=w850, "Boolean"=w848, "Boolean"=w846) -> (w875:T7)  [unwired: 1 in]
            n511 = local write "PARAMETERS VIDEO"(w875) -> ()
          }
          frame True {
          }
        }
      }
      frame #1 {
        n512 = case shown="True" FALSE {
          frame False {
          }
          frame True {
            n513 = while {
              stop <- "Play Button" stop-if-true
              "Индикатор камеры" <- FALSE ("Индикатор камеры")
            }
          }
        }
      }
      frame #2 {
        w906 = T8 4 items=["Grayscale (U8)", "Grayscale (I16)", "Grayscale (SGL)", "Complex (CSG)", "RGB (U32)", "HSL (U32)", "RGB (U64)", "Grayscale (U16)"] ("Image Type")
        w911 = T8 4 items=["Grayscale (U8)", "Grayscale (I16)", "Grayscale (SGL)", "Complex (CSG)", "RGB (U32)", "HSL (U32)", "RGB (U64)", "Grayscale (U16)"] ("Image Type")
        n514 = call <vilib>:"IMAQdx Open Camera.vi"("Session In"="CAM") -> ("Session Out"=w913:T1)  [unwired: 9 in, 1 out]
        n515 = call <vilib>:"IMAQdx Configure Grab.vi"("Session In"=w913) -> ("Session Out"=w909:T1)  [unwired: 9 in, 1 out]
        n516 = call "IMAQ Create"("Image Name"="capture", "Image Type"=w911) -> ("New Image"=w908:T4)  [unwired: 3 in, 1 out]
        n517 = call "IMAQ Create"("Image Name"="capture2", "Image Type"=w906) -> ("New Image"=w905:T4)  [unwired: 3 in, 1 out]
        n518 = while {
          tunnel: [w928] -> w914
          tunnel: w909 -> [w918]
          tunnel: w908 -> [w917]
          tunnel: w905 -> [w915]
          stop <- "Media Stop Button" stop-if-true
          n519 = flat-sequence {
            tunnel: [w932] -> w927
            tunnel: [w929] -> w925
            tunnel: w918 -> [w931]
            tunnel: w917 -> [w930]
            tunnel: [w929] -> w916
            tunnel: w927 -> [w941]
            tunnel: [w941] -> w926
            tunnel: w925 -> [w940]
            tunnel: [w940] -> w924
            tunnel: w916 -> [w939]
            tunnel: w915 -> [w935]
            tunnel: w926 -> [w961]
            tunnel: w924 -> [w960]
            tunnel: [w961] -> w923
            tunnel: [w959] -> w920
            tunnel: w923 -> [w983]
            tunnel: [w983] -> w922
            tunnel: [w982] -> w921
            tunnel: w920 -> [w982]
            tunnel: [w985] -> w928
            tunnel: w922 -> [w985]
            tunnel: w921 -> [w984]
            frame #0 {
              n520 = local write "Индикатор камеры"(TRUE ("Индикатор камеры")) -> ()
              n521 = call <vilib>:"IMAQdx Grab.vi"("Image In"=w930, "Session In"=w931) -> ("Image Out"=w929:T4, "Session Out"=w932:T1)  [unwired: 6 in, 2 out]
            }
            frame #1 {
              w934 = u32 1 items=["Horizontal", "Vertical", "Central", "1st Diagonal", "2nd Diagonal"] ("Type of Symmetry")
              n522 = call "IMAQ Copy"("Image Dst"=w935, "Image Src"=w939) -> ("Image Dst Out"=w937:T4)  [unwired: 4 in, 1 out]
              n523 = call "IMAQ Symmetry"("Type of Symmetry"=w934, "Image Dst"=w935, "Image Src"=w937) -> ("Image Dst Out"=w936:T4)  [unwired: 2 in, 1 out]
              n524 = call-poly "IMAQ Write File 2"("File Path"=path "D:/image", "Image"=w936) -> ()  [unwired: 8 in, 2 out]
            }
            frame #2 {
              (unwired) 7 items=["Red", "Green", "Blue", "Hue", "Saturation", "Luminance", "Value", "Intensity"] ("Color Plane")
              (unwired) u32 8487297 ("Color Box")
              (unwired) 612
              n525 = Wait (ms)(milliseconds to wait="DELAY") -> ()  [unwired: 1 out]
              n526 = Increment(x="Numeric") -> (x+1=w962:i16)
              n527 = local write "Numeric"(w962) -> ()
              n528 = call "IMAQ Subtract"("Image Src A"=w960, "Constant"="CALIBRATION") -> ("Image Dst Out"=w970:T4)  [unwired: 5 in, 1 out]
              n529 = call "IMAQ ExtractSingleColorPlane"("Color Plane"="SHEMA", "Image Src"=w970) -> ("Image Dst Out"=w949:T4)  [unwired: 8 in, 1 out]
              n530 = Unbundle("HOOK") -> ("Top"=w946:i32, "Bottom"=w945:i32)  [unwired: 3 out]
              n531 = Greater?(x=w946, y=w945) -> (0:w948:bool)
              n532 = case shown="True" "Blank Button" {
                tunnel: w949 -> [w977 w981]
                tunnel: [w977 w980] -> w956
                frame False {
                }
                frame True {
                  (unwired) cluster{"Lower value":sgl, "Upper value":sgl} {"Lower value"=124.0, "Upper value"=255.0} ("Range")
                  (unwired) u32 16448250 ("Color Box 2")
                  n533 = call "IMAQ Threshold"("Replace Value"="WORK COLOR", "Range"="BINAR LEVEL", "Image Src"=w981) -> ("Image Dst Out"=w980:T4)  [unwired: 3 in, 5 out]
                }
              }
              n534 = case shown="False" w948 {
                tunnel: [w974 w976] -> w947
                tunnel: w946 -> [w973 w976]
                tunnel: w945 -> [w974 w975]
                tunnel: [w973 w975] -> w944
                frame False {
                }
                frame True {
                }
              }
              n535 = Subtract(x=w947, y=w944) -> (x-y=w954:i32)
              n536 = Multiply(x="D, заготовки", y=i16 10) -> (x*y=w951:i16)
              n537 = Divide(x=w951, y=w954) -> (x/y=w950:dbl)
              "x/y" <- w950
              n538 = call "IMAQ Clamp Horizontal Max"("Settings"="PARAMETERS VIDEO", "Rectangle"="HOOK", "Image"=w956) -> ("Distance"=w968:sgl, "Image Out"=w959:T4)  [unwired: 4 in, 3 out]
              "Distance зазор" <- w968
              n539 = Multiply(x=w968, y=w950) -> (x*y=w966:dbl)
              "x*y" <- w966
              n540 = Divide(x=w966, y=10.0) -> (x/y=w964:dbl)
              n541 = Divide(x=800, y=574) -> ()  [unwired: 1 out]
              n542 = To Word Integer(number=w964) -> (16bit integer=→"16bit integer":i16)
              "Индикатор камеры 2" <- "Blank Button"
            }
            frame #3 {
            }
            frame #4 {
              "индикация видео" <- w984
            }
          }
        }
      }
    }
    n543 = Wait Until Next ms Multiple(millisecond multiple=u32 10) -> ()  [unwired: 1 out]
    n544 = call <vilib>:"IMAQdx Close Camera.vi"("Session In"=w821) -> ()  [unwired: 10 in, 1 out]
  }
